vi "Live Capture Functional Stack.7.64bit.vi"() -> ()   [LabVIEW 2014]
uses:
  subvis/Stack Track.ctl
  subvis/Stack_State.ctl
  CameraControlTypeDef.ctl
  Desktop/camtiff/ctiff.llb/__CTIFFNewFileAndStyleUINT16.vi
  Desktop/camtiff/ctiff.llb/__CTIFFAddNewPageUINT16.vi
panel:
  in  "Capture Mode":bool
  out "Record Ready":bool
  in  "Stacks":dbl=1.0
  in  "Time Lapse":bool
  out "Stack Frames":i32=100
  in  "Stack Frames":i32=100
  in  "Temp":path=path "C:/temp.tmp"
  in  "Frames":i32=100
  in  "HardDisk Record":bool
  in  "Internal Line Interval":dbl
  in  "Slit Width / Lines":sgl=150.0
  in  "Camera Readout Mode":u16(ring)=12 items=["Full Frame"=1, "Slit Scanning"=12]
  in  "Readout Direction":sgl(ring)=1.0 items=["Forward"=1, "Backward"=2]
  in  "Trigger Mode":sgl(ring)=1.0 items=["Normal"=1, "Start "=6]
  in  "Trigger Source":sgl(ring)=2.0 items=["Internal"=1, "External"=2]
  out "State":T1=enum."Start Sequence"
  out "Image":u16[][](graph)
  out "Saving":bool
  in  "AutoIncrement":bool=TRUE
  in  "Path":path=path "C:/Users/spim/Desktop/Craig Cap/temp/a.tiff"
  in  "Frames":i32=100
  out "Frame Index":i32
  out "error out":errorcluster
  in  "stop":bool
  in  "Ram Record":bool
  out "Total Frames":i32
  out "Elapsed Time":u32
  out "Software FPS":dbl
  out "Camera FPS":dbl
  in  "H Offset":i32 min=0 max=0 step=4
  in  "H Width":i32 min=0 max=2048 step=4
  out "SMD":dbl
  out "SHO":i32
  in  "V Offset":i32 min=0 max=0 step=4
  in  "V Width":i32 min=0 max=2048 step=4
  in  "Binning":u16(ring) items=["1x1"=1, "2x2"=2, "4x4"=4]
  out "SHW":i32
  out "SVO":i32
  out "SVW":i32
  in  "Scan Mode":dbl min=0.0 max=2.0 step=1.0
  in  "Exposure":dbl min=0.0 max=10.000004210526315 step=1e-08
  out "EXP":dbl
  out "Camera Model":string
  out "Camera Version":string
  out "Camera Serial":string
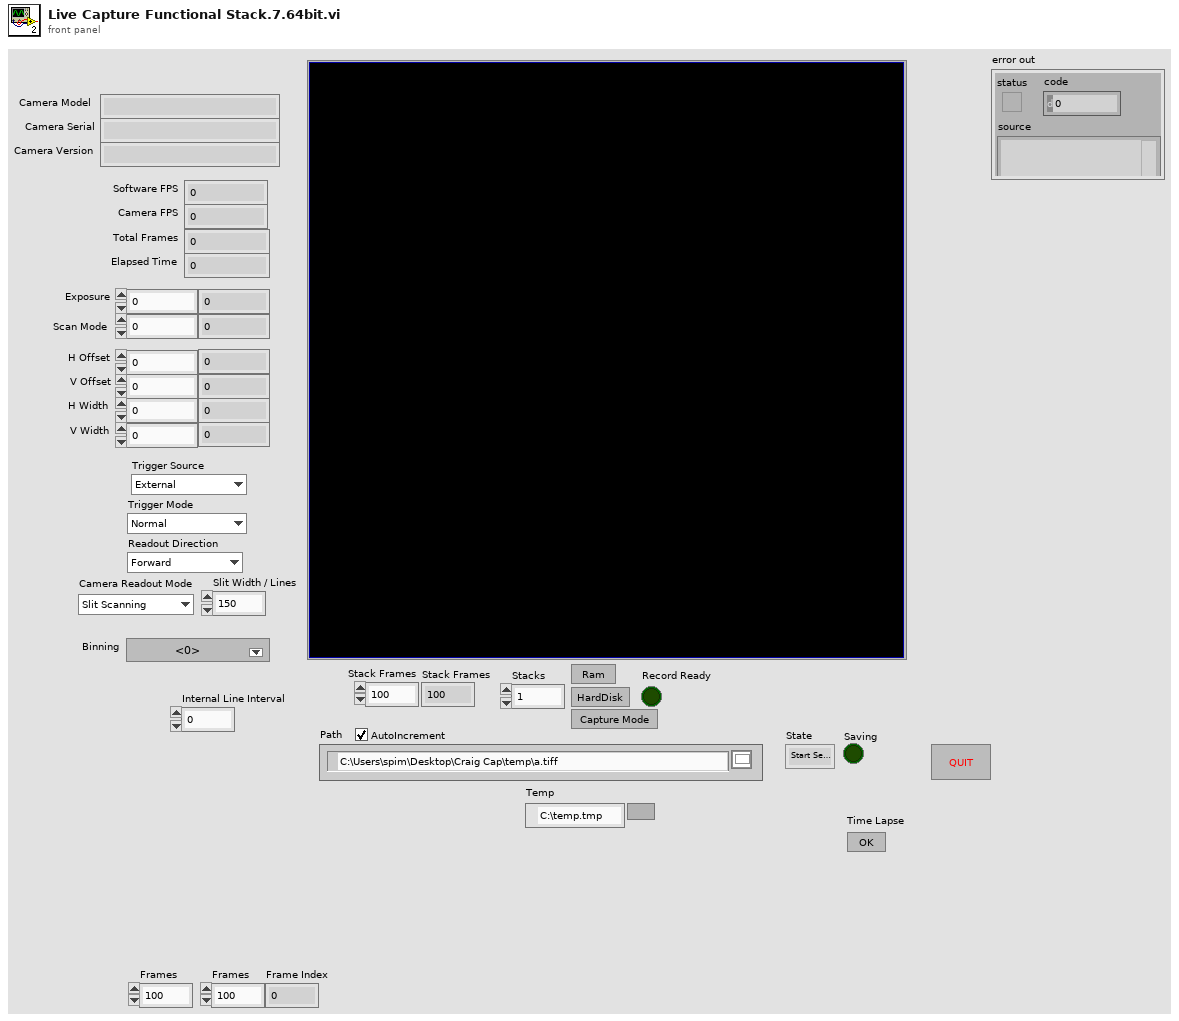
[diagram p1: front panel]
types:
  T1 = typedef "Stack Track.ctl" = enum16{"Idle", "Start Sequence", "Read Disk", "STOP", "Collecting", "End"}
  T2 = typedef "CameraControlTypeDef.ctl" = enum16{"IntervalLineInt", "Ram Record", "HardDisk Record", "Disengage Update", "Update", "Idle", "ROI", "Binning", "Scan Mode", "Trigger Mode", "Readout Mode", "Readout Direction", "Preview"}
  T3 = typedef "Stack_State.ctl" = cluster{"State":T1, "Stack Number":i32, "Image":u16[][], "Stacks":i32}
  T4 = enum8{"Enabled", "Disabled", "Disabled and Grayed Out"}
  T5 = cluster{"Model":string, "Camera ID":string, "Firmware":string}
  T6 = cluster{"Value":i32, "Minimum":i32, "Maximum":i32, "Increment":i32}
  T7 = cluster{"height":u32, "width":u32, "datatype":u32}
  T8 = cluster{"H Offset":i32, "V Offset":i32, "H Width":i32, "V Width":i32}
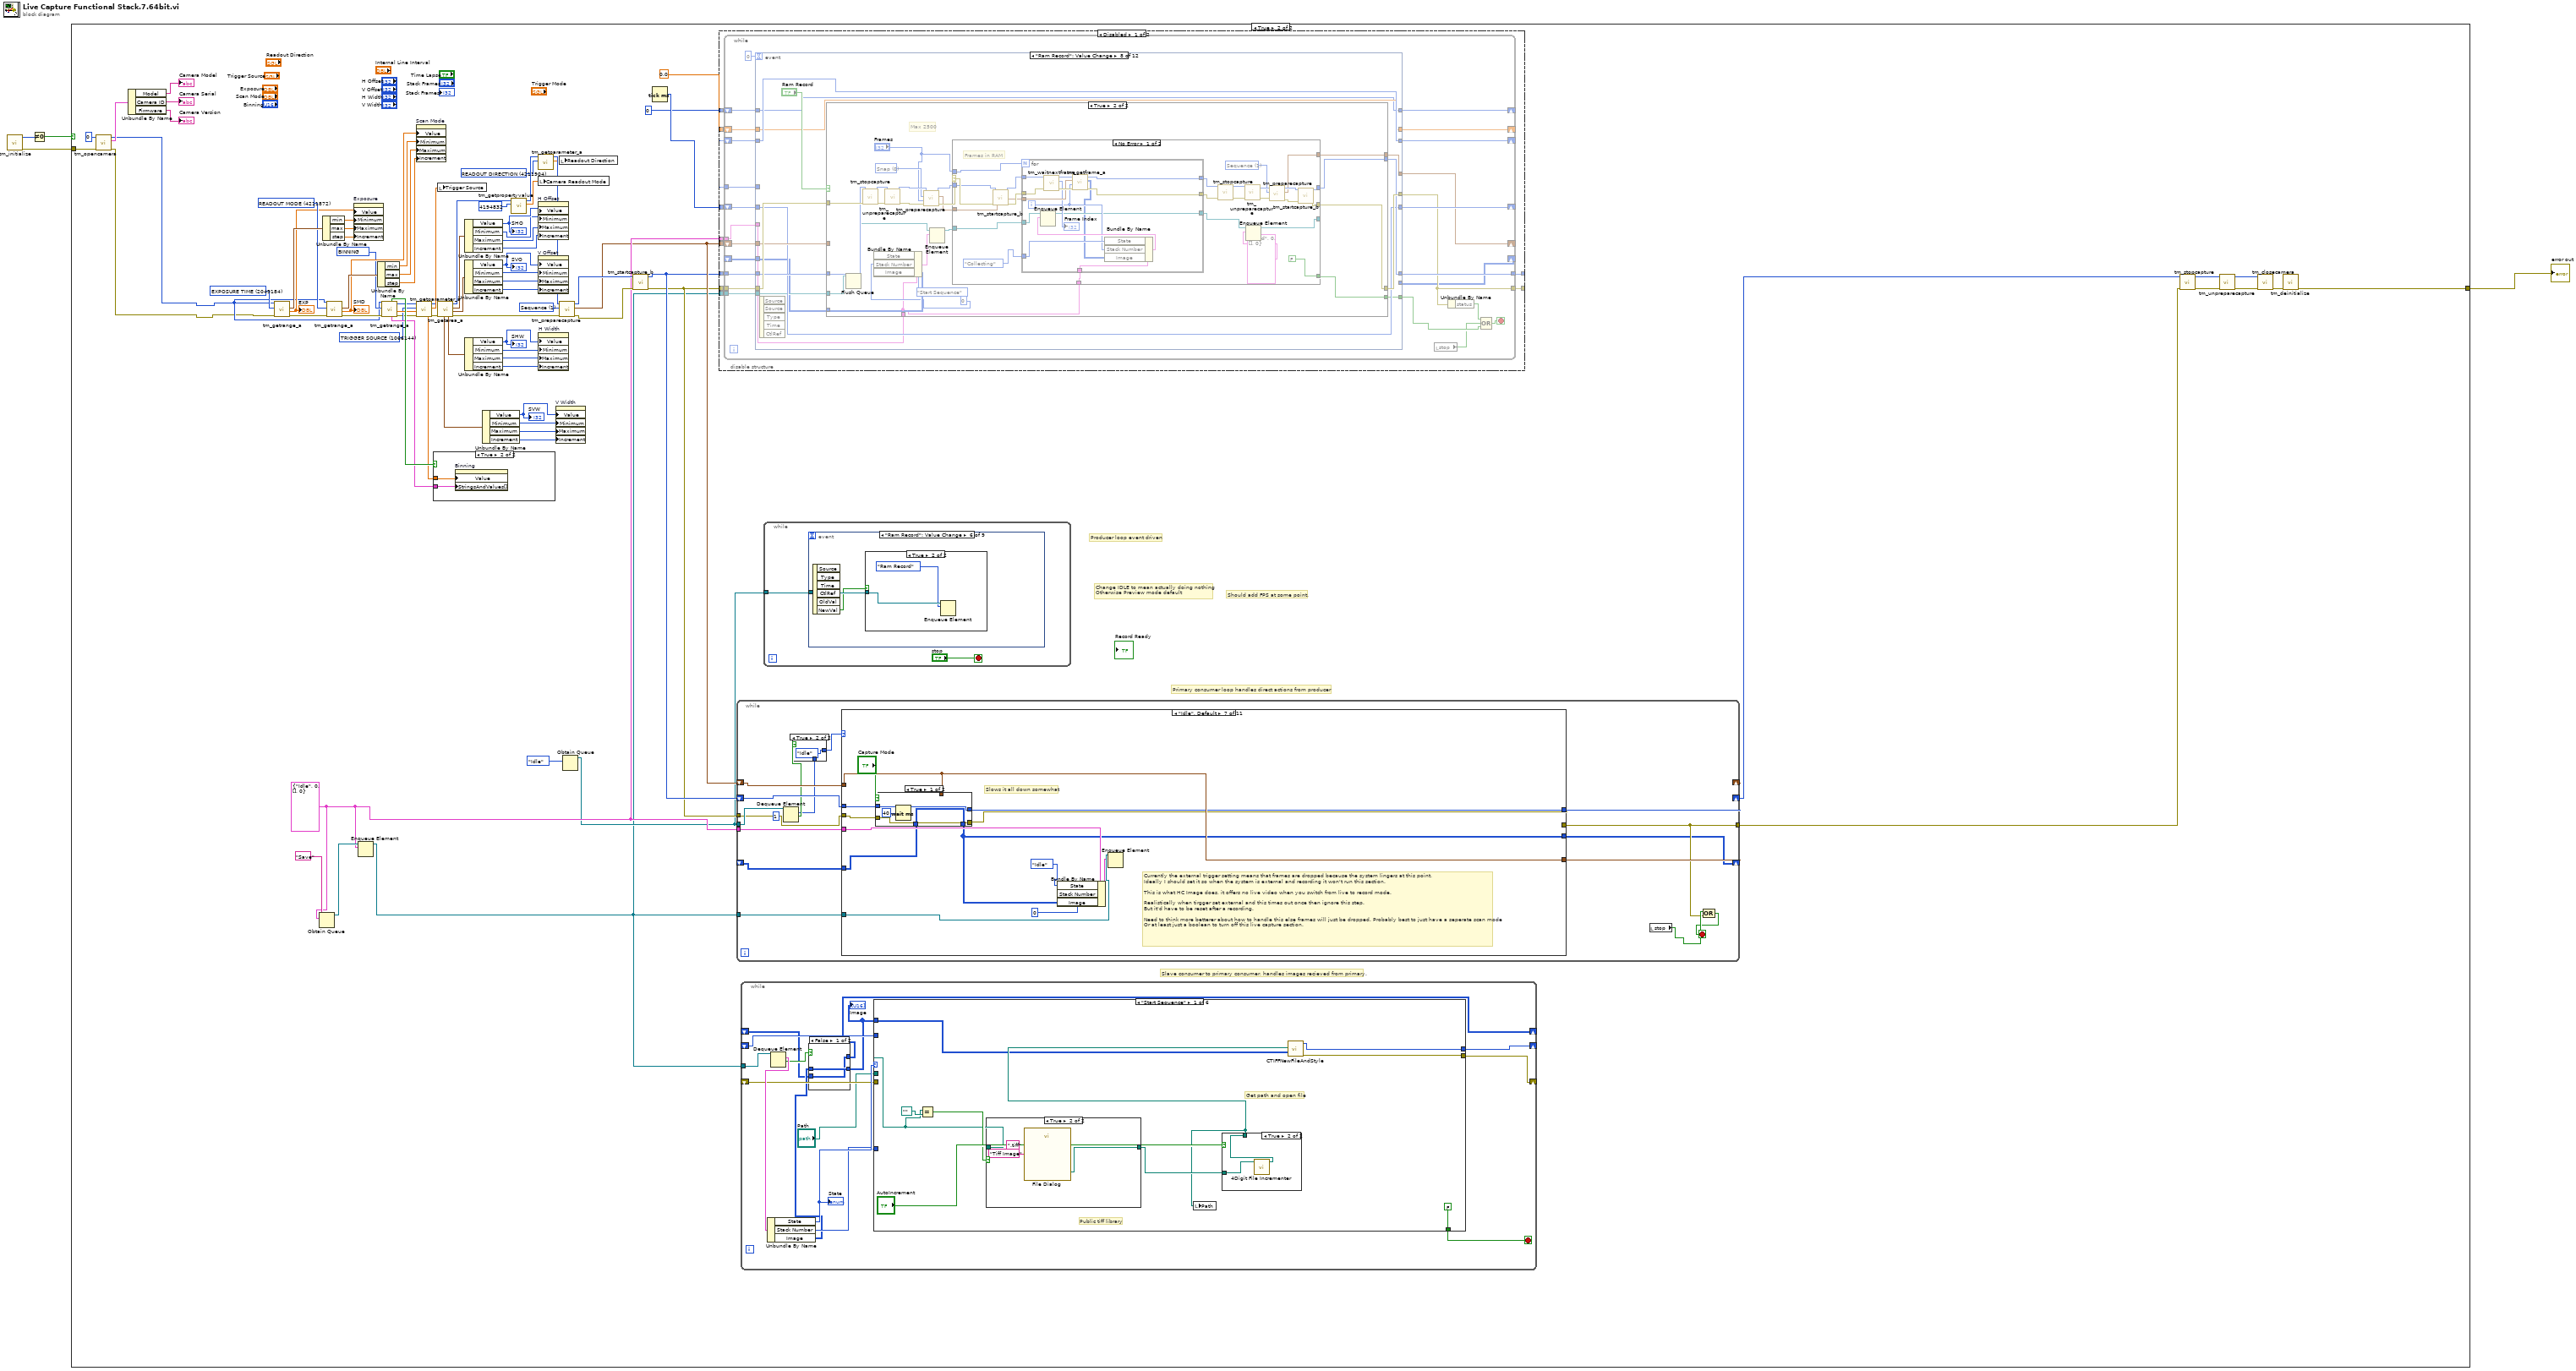
[diagram p0: block diagram]
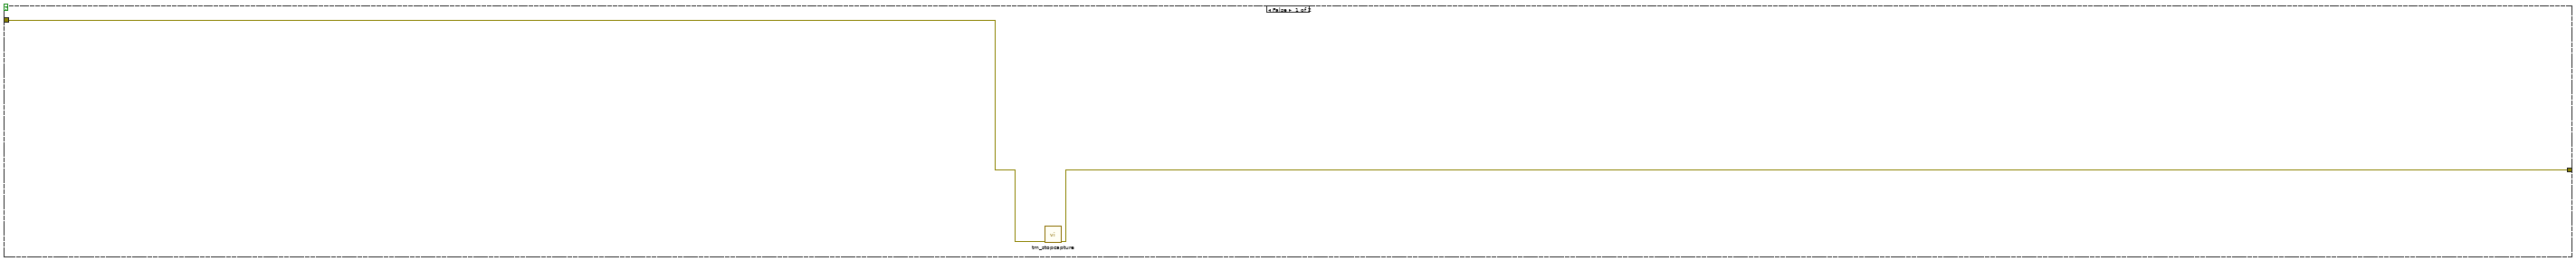
[diagram p2: hidden frame]
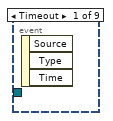
[diagram p3: hidden frame]
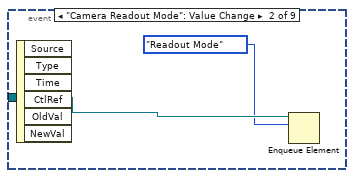
[diagram p4: hidden frame]
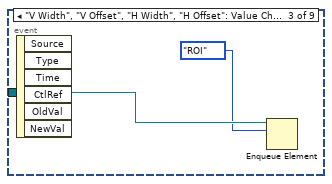
[diagram p5: hidden frame]
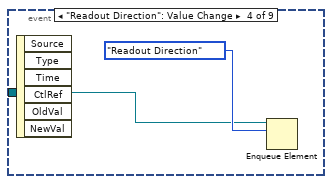
[diagram p6: hidden frame]
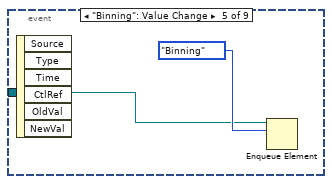
[diagram p7: hidden frame]
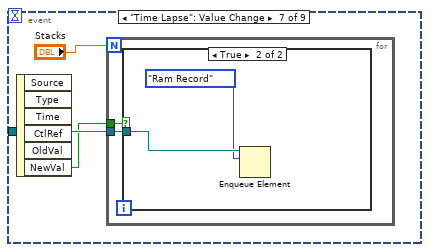
[diagram p9: hidden frame]
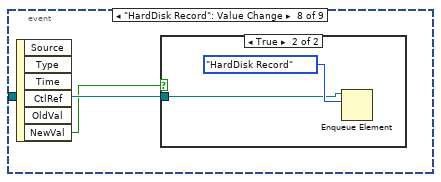
[diagram p11: hidden frame]
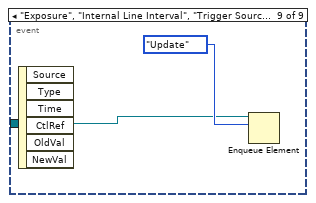
[diagram p13: hidden frame]
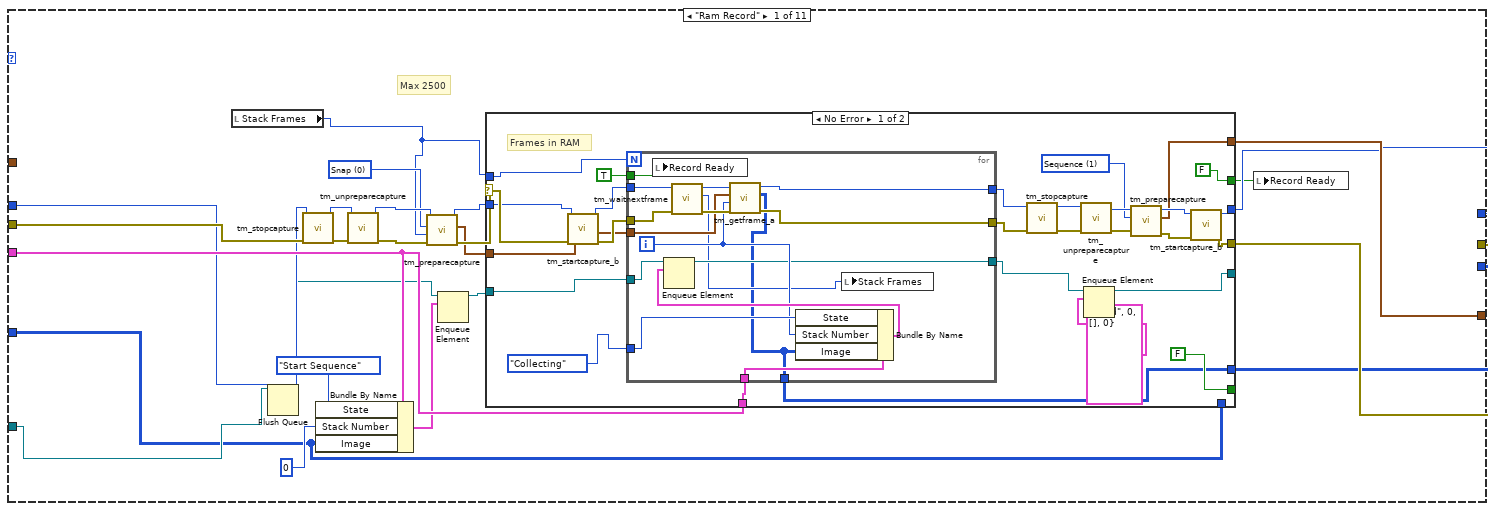
[diagram p15: hidden frame]
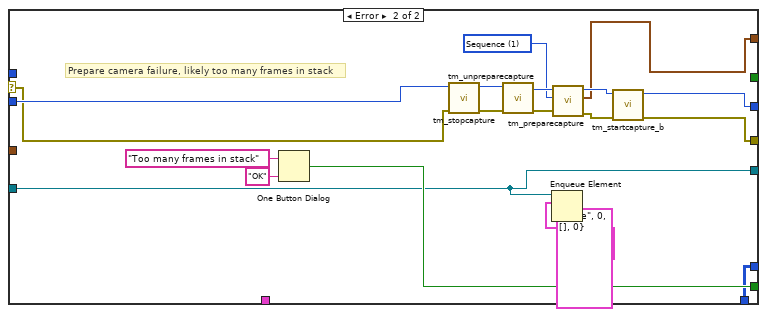
[diagram p16: hidden frame]
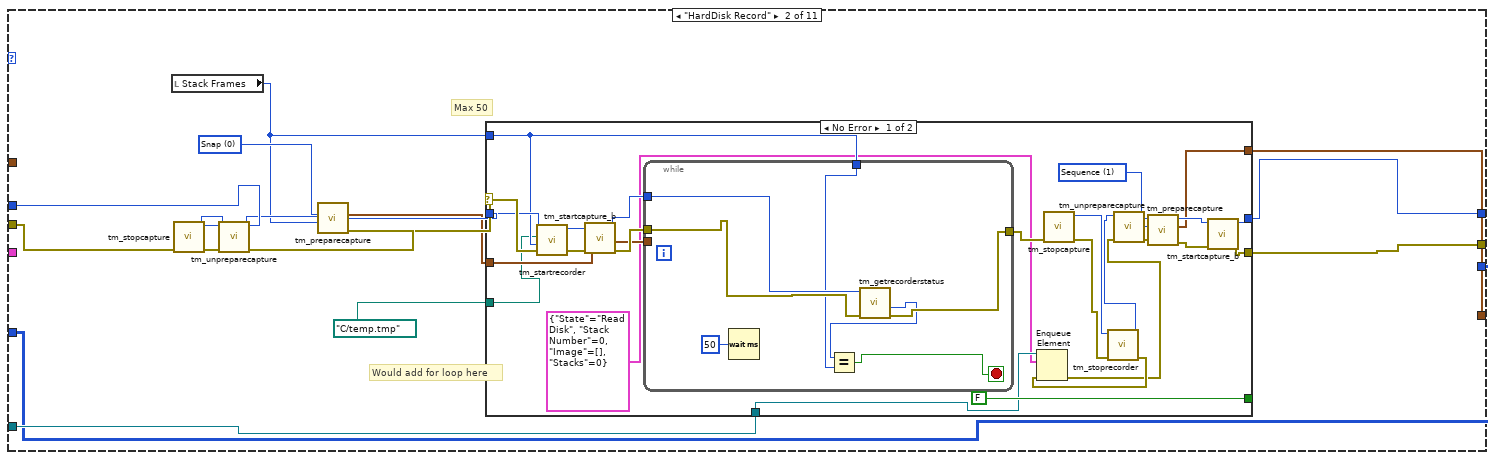
[diagram p17: hidden frame]
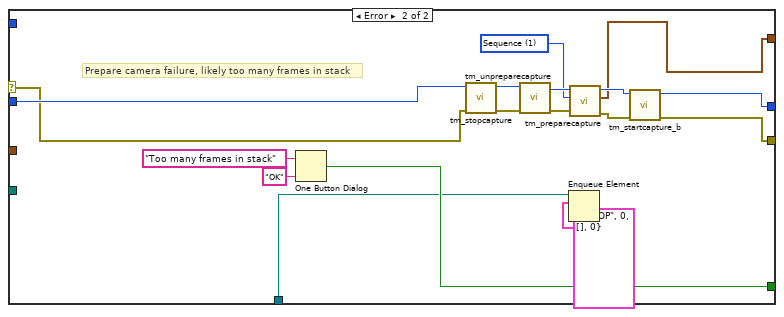
[diagram p18: hidden frame]
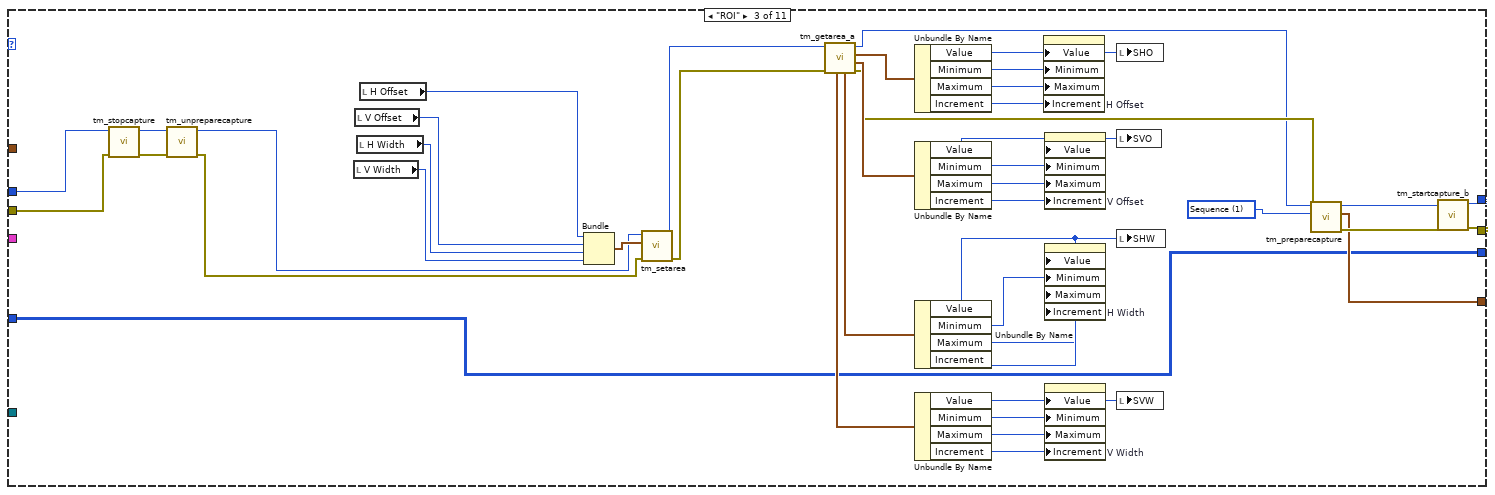
[diagram p19: hidden frame]
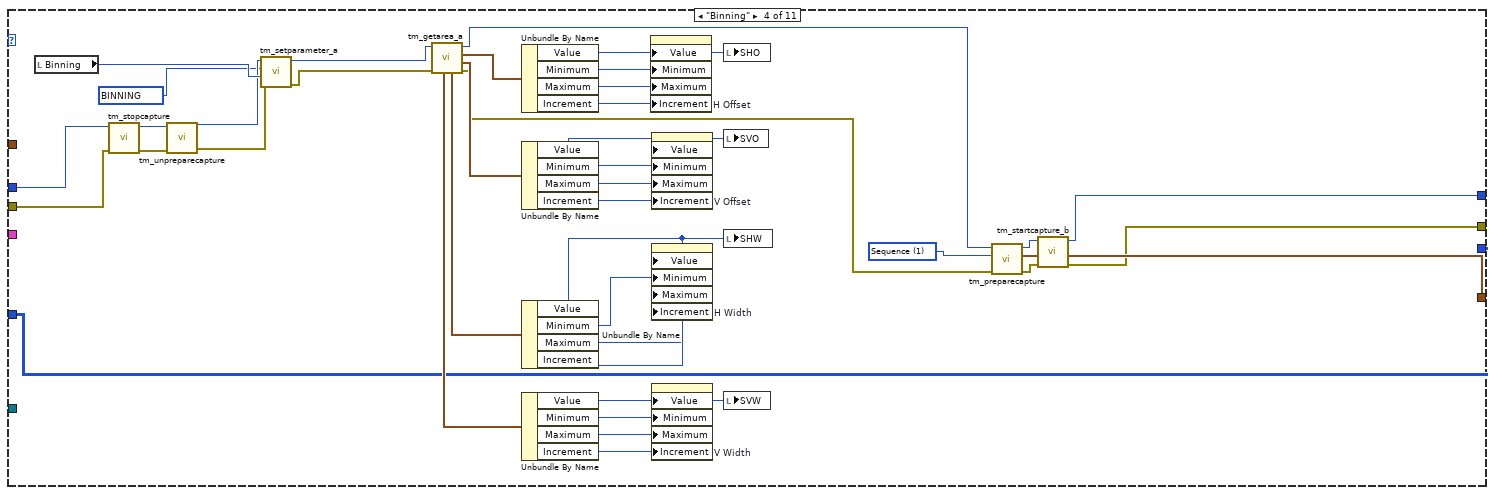
[diagram p20: hidden frame]
diagram:
  n1 = call <userlib>:"tm_initialize.vi"() -> ("error out"=w2:errorcluster, "Number Of Cameras"=w1:u32)  [unwired: 8 in, 2 out]
  n2 = Not Equal To 0?(x=w1) -> (x != 0?=w4:bool)
  n3 = case shown="True" w4 {
    tunnel: [w5 w86] -> w3
    tunnel: w2 -> [w6 w89]
    frame False {
      n4 = call <userlib>:"tm_stopcapture.vi"("error in (no error)"=w6) -> ("error out"=w5:errorcluster)  [unwired: 9 in, 1 out]
    }
    frame True {
      w22 = u32 4211904 items=["SENSOR MODE"=4212128, "CCD MODE"=4212384, "READOUT MODE"=4211872, "ACTIVE VIEW INDEX"=4343136, "BITS PER CHANNEL"=4342976, "IMAGE PIXEL TYPE"=4343296, "BINNING"=4215968, "EXPOSURE TIME"=2049184, "CONTRAST GAIN"=3163312, "CONTRAST OFFSET"=3163328, "LIGHT MODE"=2114720, "SENSITIVITY"=2114992, "PHOTON IMAGING MODE"=2115200, "HIGH DYNAMIC RANGE MODE"=3163360, "WHITE BALANCE"=3163568, "TEMPERATURE"=2115232, "TEMPERATURE TARGET"=2115264, "SENSOR COOLER FAN"=2115296, "LINEBUNDLE HEIGHT"=4212192, "MECHANICAL SHUTTER"=2115488, "BACK FOCUS POSITION"=8422304, "TRIGGER CONNECTOR"=1066432, "TRIGGER SOURCE"=1066144, "OUTPUT TRIGGER SOURCE"=1852576, "TRIGGER GLOBAL EXPOSURE"=2049680, "FIRST TRIGGER BEHAVIOR"=2049696, "CHANNEL SYNC"=1852352, "READOUT DIRECTION"=4211904, "PRE HSYNC COUNT"=1852704] ("Parameter")
      w32 = u32 1066144 items=["SENSOR MODE"=4212128, "CCD MODE"=4212384, "READOUT MODE"=4211872, "ACTIVE VIEW INDEX"=4343136, "BITS PER CHANNEL"=4342976, "IMAGE PIXEL TYPE"=4343296, "BINNING"=4215968, "EXPOSURE TIME"=2049184, "CONTRAST GAIN"=3163312, "CONTRAST OFFSET"=3163328, "LIGHT MODE"=2114720, "SENSITIVITY"=2114992, "PHOTON IMAGING MODE"=2115200, "HIGH DYNAMIC RANGE MODE"=3163360, "WHITE BALANCE"=3163568, "TEMPERATURE"=2115232, "TEMPERATURE TARGET"=2115264, "SENSOR COOLER FAN"=2115296, "LINEBUNDLE HEIGHT"=4212192, "MECHANICAL SHUTTER"=2115488, "BACK FOCUS POSITION"=8422304, "TRIGGER CONNECTOR"=1066432, "TRIGGER SOURCE"=1066144, "OUTPUT TRIGGER SOURCE"=1852576, "TRIGGER GLOBAL EXPOSURE"=2049680, "FIRST TRIGGER BEHAVIOR"=2049696, "CHANNEL SYNC"=1852352, "READOUT DIRECTION"=4211904, "PRE HSYNC COUNT"=1852704] ("Parameter")
      w15 = T3 {"State"=enum."Idle", "Stack Number"=0, "Image"=[], "Stacks"=0} ("input cluster")
      w37 = u32 2049184 items=["BINNING"=4215968, "BITS PER CHANNEL"=4342976, "ACTIVE VIEW INDEX"=4343136, "CCD MODE"=4212384, "SENSOR MODE"=4212128, "READOUT MODE"=4211872, "EXPOSURE TIME"=2049184, "CONTRAST GAIN"=3163312, "CONTRAST OFFSET"=3163328, "LIGHT MODE"=2114720, "SENSITIVITY"=2114992, "WHITE BALANCE"=3163568, "PHOTON IMAGING MODE"=2115200, "HIGH DYNAMIC RANGE MODE"=3163360, "TRIGGER SOURCE"=1066144, "TRIGGER ACTIVE"=1066160, "TRIGGER MODE"=1066400, "TRIGGER POLARITY"=1066416, "TRIGGER GLOBAL EXPOSURE"=2049680, "FIRST TRIGGER BEHAVIOR"=2049696, "TRIGGER TIMES"=1066448, "OUTPUT TRIGGER POLARITY"=1852592, "OUTPUT TRIGGER DELAY"=1852624, "OUTPUT TRIGGER PERIOD"=1852640, "TEMPERATURE"=2115232, "TEMPERATURE TARGET"=2115264, "SENSOR COOLER FAN"=2115296, "MECHANICAL SHUTTER"=2115488, "BACK FOCUS POSITION"=8422304, "FRAMEBUNDLE MODE"=4346784, "FRAMEBUNDLE NUMBER"=4346800, "LINEBUNDLE HEIGHT"=4212192, "TRIGGER CONNECTOR"=1066432, "IMAGE PIXEL TYPE"=4343296, "OUTPUT TRIGGER KIND"=1852656, "READOUT DIRECTION"=4211904, "CHANNEL SYNC"=1852352] ("Parameter")
      w38 = u32 4211872 items=["BINNING"=4215968, "BITS PER CHANNEL"=4342976, "ACTIVE VIEW INDEX"=4343136, "CCD MODE"=4212384, "SENSOR MODE"=4212128, "READOUT MODE"=4211872, "EXPOSURE TIME"=2049184, "CONTRAST GAIN"=3163312, "CONTRAST OFFSET"=3163328, "LIGHT MODE"=2114720, "SENSITIVITY"=2114992, "WHITE BALANCE"=3163568, "PHOTON IMAGING MODE"=2115200, "HIGH DYNAMIC RANGE MODE"=3163360, "TRIGGER SOURCE"=1066144, "TRIGGER ACTIVE"=1066160, "TRIGGER MODE"=1066400, "TRIGGER POLARITY"=1066416, "TRIGGER GLOBAL EXPOSURE"=2049680, "FIRST TRIGGER BEHAVIOR"=2049696, "TRIGGER TIMES"=1066448, "OUTPUT TRIGGER POLARITY"=1852592, "OUTPUT TRIGGER DELAY"=1852624, "OUTPUT TRIGGER PERIOD"=1852640, "TEMPERATURE"=2115232, "TEMPERATURE TARGET"=2115264, "SENSOR COOLER FAN"=2115296, "MECHANICAL SHUTTER"=2115488, "BACK FOCUS POSITION"=8422304, "FRAMEBUNDLE MODE"=4346784, "FRAMEBUNDLE NUMBER"=4346800, "LINEBUNDLE HEIGHT"=4212192, "TRIGGER CONNECTOR"=1066432, "IMAGE PIXEL TYPE"=4343296, "OUTPUT TRIGGER KIND"=1852656, "READOUT DIRECTION"=4211904, "CHANNEL SYNC"=1852352] ("Parameter")
      w39 = u32 4215968 items=["BINNING"=4215968, "BITS PER CHANNEL"=4342976, "ACTIVE VIEW INDEX"=4343136, "CCD MODE"=4212384, "SENSOR MODE"=4212128, "READOUT MODE"=4211872, "EXPOSURE TIME"=2049184, "CONTRAST GAIN"=3163312, "CONTRAST OFFSET"=3163328, "LIGHT MODE"=2114720, "SENSITIVITY"=2114992, "WHITE BALANCE"=3163568, "PHOTON IMAGING MODE"=2115200, "HIGH DYNAMIC RANGE MODE"=3163360, "TRIGGER SOURCE"=1066144, "TRIGGER ACTIVE"=1066160, "TRIGGER MODE"=1066400, "TRIGGER POLARITY"=1066416, "TRIGGER GLOBAL EXPOSURE"=2049680, "FIRST TRIGGER BEHAVIOR"=2049696, "TRIGGER TIMES"=1066448, "OUTPUT TRIGGER POLARITY"=1852592, "OUTPUT TRIGGER DELAY"=1852624, "OUTPUT TRIGGER PERIOD"=1852640, "TEMPERATURE"=2115232, "TEMPERATURE TARGET"=2115264, "SENSOR COOLER FAN"=2115296, "MECHANICAL SHUTTER"=2115488, "BACK FOCUS POSITION"=8422304, "FRAMEBUNDLE MODE"=4346784, "FRAMEBUNDLE NUMBER"=4346800, "LINEBUNDLE HEIGHT"=4212192, "TRIGGER CONNECTOR"=1066432, "IMAGE PIXEL TYPE"=4343296, "OUTPUT TRIGGER KIND"=1852656, "READOUT DIRECTION"=4211904, "CHANNEL SYNC"=1852352] ("Parameter")
      w84 = 1 items=["Snap", "Sequence"] ("Capture mode")
      # "Change IDLE to mean actually doing nothing\nOtherwise Preview mode default"
      # "Slave consumer to primary consumer, handles images recieved from primary."
      # "Primary consumer loop handles direct actions from producer"
      # "Producer loop event driven"
      # "Should add FPS at some point."
      n5 = call <userlib>:"tm_opencamera.vi"("error in (no error)"=w89, "Camera Index"=u32 0) -> ("error out"=w16:errorcluster, "Camera Details"=w51:T5, "Handle out"=w17:u32)  [unwired: 7 in]
      n6 = Unbundle By Name(w51) -> ("Model"=→"Camera Model":string, "Camera ID"=→"Camera Serial":string, "Firmware"=→"Camera Version":string)
      n7 = call <userlib>:"tm_getrange_a.vi"("error in (no error)"=w16, "Parameter"=w37, "Handle in"=w17) -> ("error out"=w46:errorcluster, "default"=w35:dbl, "Range"=w47:cluster{"min":dbl, "max":dbl, "step":dbl})  [unwired: 2 in, 4 out]
      "EXP" <- w35
      n8 = Obtain Queue(name (unnamed)="Save", element data type=w15) -> (queue out=w19:refnum<queue>)  [unwired: 3 in, 2 out]
      n9 = Unbundle By Name(w47) -> ("min"=w82:dbl, "max"=w81:dbl, "step"=w80:dbl)
      n10 = call <userlib>:"tm_getrange_a.vi"("error in (no error)"=w46, "Parameter"=w38, "Handle in"=w17) -> ("error out"=w43:errorcluster, "default"=w44:dbl, "Range"=w45:cluster{"min":dbl, "max":dbl, "step":dbl})  [unwired: 2 in, 4 out]
      "SMD" <- w44
      n11 = property on="Exposure" class="DigNum (strict)"("Value"=w35, "Minimum"=w82, "Maximum"=w81, "Increment"=w80) -> ()  [unwired: 2 in, 2 out]
      n12 = Enqueue Element(queue=w19, element=w15) -> (queue out=w9:refnum<queue>)  [unwired: 2 in, 2 out]
      n13 = Unbundle By Name(w45) -> ("min"=w79:dbl, "max"=w78:dbl, "step"=w77:dbl)
      n14 = call <userlib>:"tm_getrange_a.vi"("error in (no error)"=w43, "Parameter"=w39, "Handle in"=w17) -> ("error out"=w29:errorcluster, "default"=w41:dbl, "Handle out"=w31:u32, "Value Names"=w40:cluster{"Name":string, "Value":dbl}[], "Writable"=w42:bool)  [unwired: 2 in, 2 out]
      n15 = property on="Scan Mode" class="DigNum (strict)"("Value"=w44, "Minimum"=w79, "Maximum"=w78, "Increment"=w77) -> ()  [unwired: 2 in, 2 out]
      n16 = call <userlib>:"tm_getparameter_a.vi"("error in (no error)"=w29, "Parameter"=w32, "Handle in"=w31) -> ("error out"=w28:errorcluster, "Value out"=w33:dbl, "Handle out"=w30:u32)  [unwired: 6 in]
      n17 = case shown="True" w42 {
        tunnel: w40 -> [_ w1109]
        tunnel: w41 -> [_ w1108]
        frame False {
        }
        frame True {
          n18 = property on="Binning" class="Ring (strict)"("Value"=w1108, "StringsAndValues[]"=w1109) -> ()  [unwired: 2 in, 2 out]
        }
      }
      n19 = local write "Trigger Source"(w33) -> ()
      n20 = call <userlib>:"tm_getarea_a.vi"("error in (no error)"=w28, "Handle in"=w30) -> ("error out"=w34:errorcluster, "V Offset"=w76:T6, "H Offset"=w57:T6, "Handle out"=w25:u32, "H Width"=w75:T6, "V Width"=w74:T6)  [unwired: 4 in]
      n21 = Unbundle By Name(w57) -> ("Value"=w56:i32, "Minimum"=w55:i32, "Maximum"=w54:i32, "Increment"=w53:i32)
      "SHO" <- w56
      n22 = Unbundle By Name(w76) -> ("Value"=w64:i32, "Minimum"=w73:i32, "Maximum"=w72:i32, "Increment"=w71:i32)
      "SVO" <- w64
      n23 = Unbundle By Name(w75) -> ("Value"=w63:i32, "Minimum"=w70:i32, "Maximum"=w69:i32, "Increment"=w68:i32)
      "SHW" <- w63
      n24 = Unbundle By Name(w74) -> ("Value"=w62:i32, "Minimum"=w67:i32, "Maximum"=w66:i32, "Increment"=w65:i32)
      "SVW" <- w62
      n25 = call <userlib>:"tm_getpropertyvalue.vi"("Property ID"=u32 4194832, "Handle in"=w25) -> ("Value in"=w26:sgl, "Handle out"=w24:u32)  [unwired: 7 in, 1 out]
      n26 = call <userlib>:"tm_getparameter_a.vi"("Parameter"=w22, "Handle in"=w24) -> ("Value out"=w21:dbl, "Handle out"=w23:u32)  [unwired: 7 in, 1 out]
      n27 = local write "Camera Readout Mode"(w26) -> ()
      n28 = property on="H Offset" class="DigNum (strict)"("Value"=w56, "Minimum"=w55, "Maximum"=w54, "Increment"=w53) -> ()  [unwired: 2 in, 2 out]
      n29 = property on="V Offset" class="DigNum (strict)"("Value"=w64, "Minimum"=w73, "Maximum"=w72, "Increment"=w71) -> ()  [unwired: 2 in, 2 out]
      n30 = property on="H Width" class="DigNum (strict)"("Value"=w63, "Minimum"=w70, "Maximum"=w69, "Increment"=w68) -> ()  [unwired: 2 in, 2 out]
      n31 = property on="V Width" class="DigNum (strict)"("Value"=w62, "Minimum"=w67, "Maximum"=w66, "Increment"=w65) -> ()  [unwired: 2 in, 2 out]
      n32 = local write "Readout Direction"(w21) -> ()
      n33 = call <userlib>:"tm_preparecapture.vi"("error in (no error)"=w34, "Capture mode"=w84, "Handle in"=w23) -> ("error out"=w18:errorcluster, "Buffer Info"=w14:T7, "Handle out"=w20:u32)  [unwired: 5 in, 1 out]
      n34 = Obtain Queue(element data type=CameraControlTypeDef."Idle" ("Enum")) -> (queue out=w10:refnum<queue>)  [unwired: 4 in, 2 out]
      n35 = call <userlib>:"tm_startcapture_b.vi"("error in (no error)"=w18, "Handle in"=w20) -> ("error out"=w12:errorcluster, "Handle out"=w13:u32)  [unwired: 8 in]
      n36 = Tick Count (ms)() -> (millisecond timer value=w83:u32)
      n37 = disable-structure shown="Disabled" {
        disable-tunnel: 0.0 -> [w525 _]
        disable-tunnel: w83 -> [w524 _]
        disable-tunnel: 0 -> [w523 _]
        disable-tunnel: [w522 _] -> _
        disable-tunnel: [w521 _] -> _
        disable-tunnel: w15 -> [w520 _]
        disable-tunnel: w14 -> [w519 _]
        disable-tunnel: w13 -> [w518 _]
        disable-tunnel: w12 -> [w517 _]
        disable-tunnel: w9 -> [w516 _]
        frame Disabled {
          n38 = while {
            tunnel: w517 -> [w539]
            tunnel: [w537] -> w521
            tunnel: [w536] -> w522
            shift-right: [w546] -> _
            shift-left: w524 -> [w544]
            shift-right: [w547] -> _
            shift-left: w525 -> [w545]
            shift-right: [w538] -> _
            shift-left: w524 -> [w542]
            tunnel: w518 -> [w540]
            tunnel: w524 -> [w543]
            shift-right: [w535] -> _
            shift-left: w519 -> [w541]
            shift-right: [w533] -> _
            shift-left: w523 -> [w534]
            tunnel: w516 -> [w532]
            shift-right: [w530] -> _
            shift-left: _ -> [w529]
            tunnel: w520 -> [w528]
            stop <- w548 stop-if-true
            n39 = event shown="[7] \"Ram Record\": Value Change" {
              selector: _ -> [_ _ _ _ _ _ _ _ _ _ _ _]
              dyn-events: _ -> [_ _ _ _ _ _ _ _ _ _ _ _]
              timeout: 0 -> [_ _ _ _ _ _ _ _ _ _ _ _]
              tunnel: [w559 w628 w642 w655 w674 w694 w716 w744 w841 w935 w971 w1016] -> w547
              tunnel: [w558 w629 w643 w656 w675 w695 w717 w745 w842 w936 w972 w1017] -> w546
              tunnel: w545 -> [w570 w628 w642 w655 w674 w694 w716 w744 w841 w935 w971 w1016]
              tunnel: w544 -> [w561 w629 w643 w656 w675 w695 w717 w745 w842 w936 w972 w1017]
              tunnel: w543 -> [w566 _ _ _ _ _ _ _ _ _ _ _]
              tunnel: w542 -> [w571 w630 w644 w657 w676 w696 w718 w740 w837 w937 w979 w1024]
              tunnel: w541 -> [w565 w627 w641 w654 _ w693 _ w741 w838 _ _ _]
              tunnel: w540 -> [w573 w623 w636 w650 w669 w687 w709 w748 w845 w932 w948 w986]
              tunnel: w539 -> [w572 w625 w632 w651 w668 w690 w708 w749 w846 w931 w947 w985]
              tunnel: [w569 w630 w644 w657 w676 w696 w718 w740 w837 w937 w979 w1024] -> w538
              tunnel: [w568 w620 w639 w647 w660 w680 w699 w746 w843 w926 w974 w1019] -> w537
              tunnel: [w567 w619 w638 w646 w659 w679 w697 w747 w844 w927 w975 w1020] -> w536
              tunnel: [w564 w627 w641 w654 w663 w693 w704 w742 w839 w925 w973 w1018] -> w535
              tunnel: w534 -> [w556 w626 w640 w653 w673 w692 w715 w743 w840 w924 w944 w980]
              tunnel: [w555 w626 w640 w653 w673 w692 w715 w743 w840 w924 w944 w980] -> w533
              tunnel: w532 -> [w550 _ _ _ _ _ _ w739 w836 _ _ _]
              tunnel: [_ _ _ _ _ _ _ w738 w835 _ _ _] -> w531
              tunnel: w528 -> [w553 _ _ _ _ _ _ w736 _ _ _ _]
              tunnel: [w552 _ _ _ _ _ _ _ _ _ _ _] -> w530
              tunnel: w529 -> [w551 _ _ _ _ _ _ w737 _ _ _ _]
              event Timeout {
                n40 = event-data() -> ()  [unwired: 1 in, 2 out]
                n41 = call <userlib>:"tm_waitnextframe.vi"("error in (no error)"=w572, "Handle in"=w573) -> ("error out"=w576:errorcluster, "Frame Count"=w557:i32, "Frame Index"=w575:i32, "Handle out"=w577:u32)  [unwired: 6 in]
                "Total Frames" <- w557
                n42 = Tick Count (ms)() -> (millisecond timer value=w563:u32)
                n43 = Increment(x=w570) -> (x+1=w560:dbl)
                n44 = Subtract(x=w563, y=w566) -> (x-y=→"Elapsed Time":u32)
                n45 = Add(x=w561, y=u32 1000) -> (x+y=w581:u32)
                n46 = Less Or Equal?(x=w581, y=w563) -> (x <= y?=w562:bool)
                n47 = Add(x=w571, y=u32 50) -> (x+y=w579:u32)
                n48 = Less Or Equal?(x=w579, y=w563) -> (x <= y?=w554:bool)
                n49 = case shown="True" w562 {
                  tunnel: w561 -> [w584 w593]
                  tunnel: [w584 w590] -> w558
                  tunnel: w560 -> [w583 w596]
                  tunnel: w563 -> [_ w590]
                  tunnel: [w583 0.0] -> w559
                  tunnel: w557 -> [_ w585]
                  tunnel: w556 -> [w582 w588]
                  tunnel: [w582 w585] -> w555
                  frame False {
                  }
                  frame True {
                    n50 = Subtract(x=w590, y=w593) -> (x-y=w592:u32)
                    n51 = Subtract(x=w585, y=w588) -> (x-y=w586:i32)
                    n52 = To Double Precision Float(number=w592) -> (double precision float=w598:dbl)
                    n53 = Divide(x=w598, y=1000.0) -> (x/y=w589:dbl)
                    n54 = To Double Precision Float(number=w586) -> (double precision float=w587:dbl)
                    n55 = Divide(x=w587, y=w589) -> (x/y=→"Camera FPS":dbl)
                    n56 = Divide(x=w596, y=w589) -> (x/y=→"Software FPS":dbl)
                  }
                }
                n57 = case shown="True" w554 {
                  tunnel: w571 -> [w603 _]
                  tunnel: w563 -> [_ w616]
                  tunnel: [w603 w616] -> w569
                  tunnel: w577 -> [w602 w615]
                  tunnel: w565 -> [w600 w610]
                  tunnel: w576 -> [w601 w614]
                  tunnel: [w602 w613] -> w568
                  tunnel: [w601 w612] -> w567
                  tunnel: w575 -> [_ w611]
                  tunnel: [w600 w610] -> w564
                  tunnel: w550 -> [_ w609]
                  tunnel: w553 -> [_ w605]
                  tunnel: [w599 w604] -> w552
                  tunnel: w551 -> [w599 _]
                  frame False {
                  }
                  frame True {
                    n58 = call <userlib>:"tm_getframe_a.vi"("error in (no error)"=w614, "Frame Index"=w611, "Buffer Info"=w610, "Handle in"=w615) -> ("error out"=w612:errorcluster, "Data 16"=w604:u16[][], "Handle out"=w613:u32)  [unwired: 3 in, 2 out]
                    n59 = Bundle By Name(cluster=w605, "State"=Stack_Track."Idle", "Stack Number"=0, "Image"=w604) -> (w606:T3)
                    n60 = Enqueue Element(queue=w609, element=w606) -> ()  [unwired: 2 in, 3 out]
                  }
                }
              }
              event "Exposure": Value Change {
                w618 = u32 2049184 items=["SENSOR MODE"=4212128, "CCD MODE"=4212384, "READOUT MODE"=4211872, "ACTIVE VIEW INDEX"=4343136, "BITS PER CHANNEL"=4342976, "IMAGE PIXEL TYPE"=4343296, "BINNING"=4215968, "EXPOSURE TIME"=2049184, "CONTRAST GAIN"=3163312, "CONTRAST OFFSET"=3163328, "LIGHT MODE"=2114720, "SENSITIVITY"=2114992, "PHOTON IMAGING MODE"=2115200, "HIGH DYNAMIC RANGE MODE"=3163360, "WHITE BALANCE"=3163568, "TEMPERATURE"=2115232, "TEMPERATURE TARGET"=2115264, "SENSOR COOLER FAN"=2115296, "LINEBUNDLE HEIGHT"=4212192, "MECHANICAL SHUTTER"=2115488, "BACK FOCUS POSITION"=8422304, "TRIGGER CONNECTOR"=1066432, "TRIGGER SOURCE"=1066144, "OUTPUT TRIGGER SOURCE"=1852576, "TRIGGER GLOBAL EXPOSURE"=2049680, "FIRST TRIGGER BEHAVIOR"=2049696, "CHANNEL SYNC"=1852352, "READOUT DIRECTION"=4211904, "PRE HSYNC COUNT"=1852704] ("Parameter")
                n61 = event-data() -> ("NewVal"=w624:dbl)  [unwired: 1 in, 2 out]
                n62 = call <userlib>:"tm_setparameter_a.vi"("error in (no error)"=w625, "Value in"=w624, "Parameter"=w618, "Handle in"=w623) -> ("error out"=w622:errorcluster, "Handle out"=w621:u32)  [unwired: 6 in]
                n63 = call <userlib>:"tm_getparameter_a.vi"("error in (no error)"=w622, "Parameter"=w618, "Handle in"=w621) -> ("error out"=w619:errorcluster, "Value out"=w617:dbl, "Handle out"=w620:u32)  [unwired: 6 in]
                n64 = local write "EXP"(w617) -> ()
              }
              event "Internal Line Interval": Value Change {
                w631 = u32 4191424 items=["SENSOR MODE"=4212128, "CCD MODE"=4212384, "READOUT MODE"=4211872, "ACTIVE VIEW INDEX"=4343136, "BITS PER CHANNEL"=4342976, "IMAGE PIXEL TYPE"=4343296, "BINNING"=4215968, "EXPOSURE TIME"=2049184, "CONTRAST GAIN"=3163312, "CONTRAST OFFSET"=3163328, "LIGHT MODE"=2114720, "SENSITIVITY"=2114992, "PHOTON IMAGING MODE"=2115200, "HIGH DYNAMIC RANGE MODE"=3163360, "WHITE BALANCE"=3163568, "TEMPERATURE"=2115232, "TEMPERATURE TARGET"=2115264, "SENSOR COOLER FAN"=2115296, "LINEBUNDLE HEIGHT"=4212192, "MECHANICAL SHUTTER"=2115488, "BACK FOCUS POSITION"=8422304, "TRIGGER CONNECTOR"=1066432, "TRIGGER SOURCE"=1066144, "OUTPUT TRIGGER SOURCE"=1852576, "TRIGGER GLOBAL EXPOSURE"=2049680, "FIRST TRIGGER BEHAVIOR"=2049696, "CHANNEL SYNC"=1852352, "READOUT DIRECTION"=4211904, "PRE HSYNC COUNT"=1852704, "INTERNAL LINE SPEED"=4191408, "INTERNAL LINE INVERVAL"=4191424] ("Parameter")
                n65 = event-data() -> ("NewVal"=w635:dbl)  [unwired: 1 in, 2 out]
                n66 = call <userlib>:"tm_setparameter_a.vi"("error in (no error)"=w632, "Value in"=w635, "Parameter"=w631, "Handle in"=w636) -> ("error out"=w633:errorcluster, "Handle out"=w634:u32)  [unwired: 6 in]
                n67 = call <userlib>:"tm_getparameter_a.vi"("error in (no error)"=w633, "Parameter"=w631, "Handle in"=w634) -> ("error out"=w638:errorcluster, "Value out"=w637:dbl, "Handle out"=w639:u32)  [unwired: 6 in]
                n68 = local write "Internal Line Interval"(w637) -> ()
              }
              event "Trigger Source": Value Change {
                w652 = u32 1066144 items=["SENSOR MODE"=4212128, "CCD MODE"=4212384, "READOUT MODE"=4211872, "ACTIVE VIEW INDEX"=4343136, "BITS PER CHANNEL"=4342976, "IMAGE PIXEL TYPE"=4343296, "BINNING"=4215968, "EXPOSURE TIME"=2049184, "CONTRAST GAIN"=3163312, "CONTRAST OFFSET"=3163328, "LIGHT MODE"=2114720, "SENSITIVITY"=2114992, "PHOTON IMAGING MODE"=2115200, "HIGH DYNAMIC RANGE MODE"=3163360, "WHITE BALANCE"=3163568, "TEMPERATURE"=2115232, "TEMPERATURE TARGET"=2115264, "SENSOR COOLER FAN"=2115296, "LINEBUNDLE HEIGHT"=4212192, "MECHANICAL SHUTTER"=2115488, "BACK FOCUS POSITION"=8422304, "TRIGGER CONNECTOR"=1066432, "TRIGGER SOURCE"=1066144, "OUTPUT TRIGGER SOURCE"=1852576, "TRIGGER GLOBAL EXPOSURE"=2049680, "FIRST TRIGGER BEHAVIOR"=2049696, "CHANNEL SYNC"=1852352, "READOUT DIRECTION"=4211904, "PRE HSYNC COUNT"=1852704] ("Parameter")
                n69 = event-data() -> ("NewVal"=w645:sgl)  [unwired: 1 in, 3 out]
                n70 = call <userlib>:"tm_setparameter_a.vi"("error in (no error)"=w651, "Value in"=w645, "Parameter"=w652, "Handle in"=w650) -> ("error out"=w649:errorcluster, "Handle out"=w648:u32)  [unwired: 6 in]
                n71 = call <userlib>:"tm_getparameter_a.vi"("error in (no error)"=w649, "Parameter"=w652, "Handle in"=w648) -> ("error out"=w646:errorcluster, "Handle out"=w647:u32)  [unwired: 6 in, 1 out]
              }
              event "Trigger Mode": Value Change {
                w664 = 1 items=["Snap", "Sequence"] ("Capture mode")
                n72 = event-data() -> ("NewVal"=w658:sgl)  [unwired: 1 in, 4 out]
                n73 = call <userlib>:"tm_stopcapture.vi"("error in (no error)"=w668, "Handle in"=w669) -> ("error out"=w671:errorcluster, "Handle out"=w670:u32)  [unwired: 8 in]
                n74 = call <userlib>:"tm_unpreparecapture.vi"("error in (no error)"=w671, "Handle in"=w670) -> ("error out"=w667:errorcluster, "Handle out"=w666:u32)  [unwired: 8 in]
                n75 = call <userlib>:"tm_setpropertyvalue.vi"("error in (no error)"=w667, "Value in"=w658, "Property ID"=u32 1049104, "Handle in"=w666) -> ("error out"=w662:errorcluster, "Handle out"=w665:u32)  [unwired: 6 in]
                n76 = call <userlib>:"tm_preparecapture.vi"("Capture mode"=w664, "Handle in"=w665) -> ("Buffer Info"=w663:T7, "Handle out"=w661:u32)  [unwired: 6 in, 2 out]
                n77 = call <userlib>:"tm_startcapture_b.vi"("error in (no error)"=w662, "Handle in"=w661) -> ("error out"=w659:errorcluster, "Handle out"=w660:u32)  [unwired: 8 in]
              }
              event "Readout Direction": Value Change {
                w685 = 1 items=["Snap", "Sequence"] ("Capture mode")
                w678 = u32 4211904 items=["SENSOR MODE"=4212128, "CCD MODE"=4212384, "READOUT MODE"=4211872, "ACTIVE VIEW INDEX"=4343136, "BITS PER CHANNEL"=4342976, "IMAGE PIXEL TYPE"=4343296, "BINNING"=4215968, "EXPOSURE TIME"=2049184, "CONTRAST GAIN"=3163312, "CONTRAST OFFSET"=3163328, "LIGHT MODE"=2114720, "SENSITIVITY"=2114992, "PHOTON IMAGING MODE"=2115200, "HIGH DYNAMIC RANGE MODE"=3163360, "WHITE BALANCE"=3163568, "TEMPERATURE"=2115232, "TEMPERATURE TARGET"=2115264, "SENSOR COOLER FAN"=2115296, "LINEBUNDLE HEIGHT"=4212192, "MECHANICAL SHUTTER"=2115488, "BACK FOCUS POSITION"=8422304, "TRIGGER CONNECTOR"=1066432, "TRIGGER SOURCE"=1066144, "OUTPUT TRIGGER SOURCE"=1852576, "TRIGGER GLOBAL EXPOSURE"=2049680, "FIRST TRIGGER BEHAVIOR"=2049696, "CHANNEL SYNC"=1852352, "READOUT DIRECTION"=4211904, "PRE HSYNC COUNT"=1852704] ("Parameter")
                n78 = event-data() -> ("NewVal"=w677:sgl)  [unwired: 1 in, 3 out]
                n79 = call <userlib>:"tm_stopcapture.vi"("error in (no error)"=w690, "Handle in"=w687) -> ("error out"=w691:errorcluster, "Handle out"=w686:u32)  [unwired: 8 in]
                n80 = call <userlib>:"tm_unpreparecapture.vi"("error in (no error)"=w691, "Handle in"=w686) -> ("error out"=w689:errorcluster, "Handle out"=w688:u32)  [unwired: 8 in]
                n81 = call <userlib>:"tm_setparameter_a.vi"("error in (no error)"=w689, "Value in"=w677, "Parameter"=w678, "Handle in"=w688) -> ("error out"=w682:errorcluster, "Handle out"=w681:u32)  [unwired: 6 in]
                n82 = call <userlib>:"tm_preparecapture.vi"("error in (no error)"=w682, "Capture mode"=w685, "Handle in"=w681) -> ("error out"=w683:errorcluster, "Handle out"=w684:u32)  [unwired: 5 in, 2 out]
                n83 = call <userlib>:"tm_startcapture_b.vi"("error in (no error)"=w683, "Handle in"=w684) -> ("error out"=w679:errorcluster, "Handle out"=w680:u32)  [unwired: 8 in]
              }
              event "Camera Readout Mode", "Slit Width / Lines": Value Change {
                w702 = 1 items=["Snap", "Sequence"] ("Capture mode")
                n84 = event-data() -> ()  [unwired: 1 in, 4 out]
                n85 = call <userlib>:"tm_stopcapture.vi"("error in (no error)"=w708, "Handle in"=w709) -> ("error out"=w710:errorcluster, "Handle out"=w706:u32)  [unwired: 8 in]
                n86 = call <userlib>:"tm_unpreparecapture.vi"("error in (no error)"=w710, "Handle in"=w706) -> ("error out"=w701:errorcluster, "Handle out"=w707:u32)  [unwired: 8 in]
                n87 = call <userlib>:"tm_setpropertyvalue.vi"("error in (no error)"=w701, "Value in"="Camera Readout Mode", "Property ID"=u32 4194832, "Handle in"=w707) -> ("error out"=w711:errorcluster, "Handle out"=w712:u32)  [unwired: 6 in]
                n88 = case shown="12" "Camera Readout Mode" {
                  tunnel: w712 -> [w723 w730]
                  tunnel: [w722 w725] -> w705
                  tunnel: w711 -> [w720 w735]
                  tunnel: [w719 w735] -> w703
                  frame 1, Default {
                    n89 = local read "Exposure"() -> (w721:dbl)
                    n90 = call <userlib>:"tm_setpropertyvalue.vi"("error in (no error)"=w720, "Value in"=w721, "Property ID"=u32 2031888, "Handle in"=w723) -> ("error out"=w719:errorcluster, "Handle out"=w722:u32)  [unwired: 6 in]
                  }
                  frame 12 {
                    n91 = local read "Exposure"() -> (w734:dbl)
                    n92 = local read "SVW"() -> (w732:i32)
                    n93 = formula code="slitExpos=frameInter*LW/(LinesToReadout\n+10+LW);\nlineInter = slitExpos / LW;"("frameInter"=w734, "LW"="Slit Width / Lines", "LinesToReadout"=w732) -> ("slitExpos"=w726:dbl, "lineInter"=w729:dbl)
                    n94 = call <userlib>:"tm_setpropertyvalue.vi"("Value in"=w729, "Property ID"=u32 4208720, "Handle in"=w730) -> ("Handle out"=w728:u32)  [unwired: 7 in, 1 out]
                    n95 = call <userlib>:"tm_setpropertyvalue.vi"("Value in"=w726, "Property ID"=u32 2031888, "Handle in"=w728) -> ("Handle out"=w725:u32)  [unwired: 7 in, 1 out]
                  }
                }
                n96 = call <userlib>:"tm_preparecapture.vi"("error in (no error)"=w703, "Capture mode"=w702, "Handle in"=w705) -> ("error out"=w698:errorcluster, "Buffer Info"=w704:T7, "Handle out"=w700:u32)  [unwired: 5 in, 1 out]
                n97 = call <userlib>:"tm_startcapture_b.vi"("error in (no error)"=w698, "Handle in"=w700) -> ("error out"=w697:errorcluster, "Handle out"=w699:u32)  [unwired: 8 in]
              }
              event "Ram Record": Value Change {
                n98 = event-data() -> ()  [unwired: 1 in, 5 out]
                n99 = case shown="True" "Ram Record" {
                  tunnel: w749 -> [w753 w776]
                  tunnel: w748 -> [w752 w773]
                  tunnel: [w753 w759] -> w747
                  tunnel: [w752 w761] -> w746
                  tunnel: [w751 w760] -> w742
                  tunnel: w741 -> [w751 _]
                  tunnel: w739 -> [_ w764]
                  tunnel: [_ w762] -> w738
                  tunnel: w737 -> [_ w758]
                  tunnel: w736 -> [_ w754]
                  frame False {
                  }
                  frame True {
                    w770 = 0 items=["Snap", "Sequence"] ("Capture mode")
                    # "Max 2500"
                    n100 = Flush Queue(queue=w764) -> (queue out=w763:refnum<queue>)  [unwired: 1 in, 2 out]
                    n101 = call <userlib>:"tm_stopcapture.vi"("error in (no error)"=w776, "Handle in"=w773) -> ("error out"=w775:errorcluster, "Handle out"=w774:u32)  [unwired: 8 in]
                    n102 = Bundle By Name(cluster=w754, "State"=Stack_Track."Start Sequence", "Stack Number"=0, "Image"=w758) -> (w755:T3)
                    n103 = call <userlib>:"tm_unpreparecapture.vi"("error in (no error)"=w775, "Handle in"=w774) -> ("error out"=w771:errorcluster, "Handle out"=w772:u32)  [unwired: 8 in]
                    n104 = call <userlib>:"tm_preparecapture.vi"("error in (no error)"=w771, "Frames"="Frames", "Capture mode"=w770, "Handle in"=w772) -> ("error out"=w769:errorcluster, "Buffer Info"=w767:T7, "Handle out"=w768:u32)  [unwired: 4 in, 1 out]
                    n105 = Enqueue Element(queue=w763, element=w755) -> (queue out=w765:refnum<queue>)  [unwired: 2 in, 2 out]
                    n106 = case shown="No Error" w769 {
                      selector: w769 -> [w801 w822]
                      tunnel: w768 -> [w800 w823]
                      tunnel: "Frames" -> [w796 _]
                      tunnel: [w781 w819] -> w761
                      tunnel: w767 -> [w797 _]
                      tunnel: [w780 w821] -> w759
                      tunnel: w765 -> [w795 w817]
                      tunnel: w754 -> [w794 _]
                      tunnel: [w779 w817] -> _
                      tunnel: [FALSE ("value") w831] -> w762
                      tunnel: [w778 w820] -> w760
                      frame No Error {
                        w786 = 1 items=["Snap", "Sequence"] ("Capture mode")
                        # "Frames in RAM"
                        n107 = call <userlib>:"tm_startcapture_b.vi"("error in (no error)"=w801, "Handle in"=w800) -> ("error out"=w798:errorcluster, "Handle out"=w799:u32)  [unwired: 8 in]
                        n108 = for {
                          N: w796 -> [_]
                          tunnel: w799 -> [w816]
                          tunnel: w798 -> [w815]
                          tunnel: w797 -> [w812]
                          tunnel: [w811] -> w792
                          tunnel: [w810] -> w791
                          tunnel: w795 -> [w808]
                          tunnel: Stack_Track."Collecting" ("Enum") -> [w806]
                          tunnel: w794 -> [w804]
                          tunnel: [w803] -> w785
                          i -> [w805]
                          n109 = call <userlib>:"tm_waitnextframe.vi"("error in (no error)"=w815, "Handle in"=w816) -> ("error out"=w813:errorcluster, "Frame Index"=→"Frame Index":i32, "Handle out"=w814:u32)  [unwired: 6 in, 1 out]
                          n110 = call <userlib>:"tm_getframe_a.vi"("error in (no error)"=w813, "Frame Index"=w805, "Buffer Info"=w812, "Handle in"=w814) -> ("error out"=w810:errorcluster, "Data 16"=w802:u16[][], "Handle out"=w811:u32)  [unwired: 3 in, 2 out]
                          n111 = Bundle By Name(cluster=w804, "State"=w806, "Stack Number"=w805, "Image"=w802) -> (w807:T3)
                          n112 = Enqueue Element(queue=w808, element=w807) -> (queue out=w803:refnum<queue>)  [unwired: 2 in, 2 out]
                        }
                        n113 = call <userlib>:"tm_stopcapture.vi"("error in (no error)"=w791, "Handle in"=w792) -> ("error out"=w789:errorcluster, "Handle out"=w790:u32)  [unwired: 8 in]
                        n114 = call <userlib>:"tm_unpreparecapture.vi"("error in (no error)"=w789, "Handle in"=w790) -> ("error out"=w788:errorcluster, "Handle out"=w787:u32)  [unwired: 8 in]
                        n115 = Enqueue Element(queue=w785, element=T3 {"State"=enum."End", "Stack Number"=0, "Image"=[], "Stacks"=0} ("input cluster")) -> (queue out=w779:refnum<queue>)  [unwired: 2 in, 2 out]
                        n116 = call <userlib>:"tm_preparecapture.vi"("error in (no error)"=w788, "Capture mode"=w786, "Handle in"=w787) -> ("error out"=w783:errorcluster, "Buffer Info"=w778:T7, "Handle out"=w782:u32)  [unwired: 5 in, 1 out]
                        n117 = call <userlib>:"tm_startcapture_b.vi"("error in (no error)"=w783, "Handle in"=w782) -> ("error out"=w780:errorcluster, "Handle out"=w781:u32)  [unwired: 8 in]
                      }
                      frame Error {
                        w826 = 1 items=["Snap", "Sequence"] ("Capture mode")
                        # "Prepare camera failure, likely too many frames in stack"
                        n118 = One Button Dialog(message="Too many frames in stack", button name ("OK")="OK") -> (true=w831:bool)
                        n119 = call <userlib>:"tm_stopcapture.vi"("error in (no error)"=w822, "Handle in"=w823) -> ("error out"=w829:errorcluster, "Handle out"=w830:u32)  [unwired: 8 in]
                        n120 = call <userlib>:"tm_unpreparecapture.vi"("error in (no error)"=w829, "Handle in"=w830) -> ("error out"=w828:errorcluster, "Handle out"=w827:u32)  [unwired: 8 in]
                        n121 = Enqueue Element(queue=w817, element=T3 {"State"=enum."Idle", "Stack Number"=0, "Image"=[], "Stacks"=0} ("input cluster")) -> ()  [unwired: 2 in, 3 out]
                        n122 = call <userlib>:"tm_preparecapture.vi"("error in (no error)"=w828, "Capture mode"=w826, "Handle in"=w827) -> ("error out"=w825:errorcluster, "Buffer Info"=w820:T7, "Handle out"=w824:u32)  [unwired: 5 in, 1 out]
                        n123 = call <userlib>:"tm_startcapture_b.vi"("error in (no error)"=w825, "Handle in"=w824) -> ("error out"=w821:errorcluster, "Handle out"=w819:u32)  [unwired: 8 in]
                      }
                    }
                  }
                }
              }
              event "HardDisk Record": Value Change {
                n124 = event-data() -> ()  [unwired: 1 in, 5 out]
                n125 = case shown="True" "HardDisk Record" {
                  tunnel: w846 -> [w849 w865]
                  tunnel: w845 -> [w848 w862]
                  tunnel: [w849 w852] -> w844
                  tunnel: [w848 w854] -> w843
                  tunnel: [w847 w853] -> w839
                  tunnel: w838 -> [w847 _]
                  tunnel: w836 -> [_ w850]
                  tunnel: [_ w855] -> w835
                  frame False {
                  }
                  frame True {
                    w859 = 0 items=["Snap", "Sequence"] ("Capture mode")
                    # "Max 50"
                    n126 = call <userlib>:"tm_stopcapture.vi"("error in (no error)"=w865, "Handle in"=w862) -> ("error out"=w864:errorcluster, "Handle out"=w863:u32)  [unwired: 8 in]
                    n127 = call <userlib>:"tm_unpreparecapture.vi"("error in (no error)"=w864, "Handle in"=w863) -> ("error out"=w860:errorcluster, "Handle out"=w861:u32)  [unwired: 8 in]
                    n128 = call <userlib>:"tm_preparecapture.vi"("error in (no error)"=w860, "Frames"="Frames", "Capture mode"=w859, "Handle in"=w861) -> ("error out"=w858:errorcluster, "Buffer Info"=w856:T7, "Handle out"=w857:u32)  [unwired: 4 in, 1 out]
                    n129 = case shown="No Error" w858 {
                      selector: w858 -> [w890 w903]
                      tunnel: w857 -> [w876 w904]
                      tunnel: [w879 w900] -> w854
                      tunnel: w856 -> [w887 _]
                      tunnel: [w878 w902] -> w852
                      tunnel: [FALSE ("value") w912] -> w855
                      tunnel: [w877 w901] -> w853
                      tunnel: "Frames" -> [w873 _]
                      tunnel: w850 -> [w867 w898]
                      frame No Error {
                        w882 = 1 items=["Snap", "Sequence"] ("Capture mode")
                        n130 = call <userlib>:"tm_startrecorder.vi"("frames"=w873, "File"="Temp", "Handle in"=w876) -> ("Handle out"=w875:u32)  [unwired: 7 in, 1 out]
                        n131 = call <userlib>:"tm_startcapture_b.vi"("error in (no error)"=w890, "Handle in"=w875) -> ("error out"=w888:errorcluster, "Handle out"=w889:u32)  [unwired: 8 in]
                        n132 = while {
                          tunnel: w889 -> [w896]
                          tunnel: w888 -> [w895]
                          tunnel: w887 -> [_]
                          tunnel: [w897] -> w885
                          tunnel: w873 -> [w892]
                          stop <- w893 stop-if-true
                          n133 = Wait (ms)(milliseconds to wait=u32 50) -> ()  [unwired: 1 out]
                          n134 = call <userlib>:"tm_getrecorderstatus.vi"("error in (no error)"=w895, "Handle"=w896) -> ("error out"=w897:errorcluster, "Count"=w891:i32)  [unwired: 6 in, 2 out]
                          n135 = Equal?(x=w891, y=w892) -> (x = y?=w893:bool)
                        }
                        n136 = call <userlib>:"tm_stopcapture.vi"("error in (no error)"=w885) -> ("error out"=w872:errorcluster, "Handle out"=w871:u32)  [unwired: 9 in]
                        n137 = call <userlib>:"tm_stoprecorder.vi"("error in (no error)"=w872, "Handle in"=w871) -> ("error out"=w869:errorcluster, "Handle out"=w870:u32)  [unwired: 8 in]
                        n138 = Enqueue Element(queue=w867, element=T3 {"State"=enum."Read Disk", "Stack Number"=0, "Image"=[], "Stacks"=0}, error in (no error)=w869) -> (error out=w868:errorcluster)  [unwired: 1 in, 2 out]
                        n139 = call <userlib>:"tm_unpreparecapture.vi"("error in (no error)"=w868, "Handle in"=w870) -> ("error out"=w884:errorcluster, "Handle out"=w883:u32)  [unwired: 8 in]
                        n140 = call <userlib>:"tm_preparecapture.vi"("error in (no error)"=w884, "Capture mode"=w882, "Handle in"=w883) -> ("error out"=w881:errorcluster, "Buffer Info"=w877:T7, "Handle out"=w880:u32)  [unwired: 5 in, 1 out]
                        n141 = call <userlib>:"tm_startcapture_b.vi"("error in (no error)"=w881, "Handle in"=w880) -> ("error out"=w878:errorcluster, "Handle out"=w879:u32)  [unwired: 8 in]
                      }
                      frame Error {
                        w907 = 1 items=["Snap", "Sequence"] ("Capture mode")
                        # "Prepare camera failure, likely too many frames in stack"
                        n142 = One Button Dialog(message="Too many frames in stack", button name ("OK")="OK") -> (true=w912:bool)
                        n143 = call <userlib>:"tm_stopcapture.vi"("error in (no error)"=w903, "Handle in"=w904) -> ("error out"=w910:errorcluster, "Handle out"=w911:u32)  [unwired: 8 in]
                        n144 = call <userlib>:"tm_unpreparecapture.vi"("error in (no error)"=w910, "Handle in"=w911) -> ("error out"=w909:errorcluster, "Handle out"=w908:u32)  [unwired: 8 in]
                        n145 = Enqueue Element(queue=w898, element=T3 {"State"=enum."STOP", "Stack Number"=0, "Image"=[], "Stacks"=0} ("input cluster")) -> ()  [unwired: 2 in, 3 out]
                        n146 = call <userlib>:"tm_preparecapture.vi"("error in (no error)"=w909, "Capture mode"=w907, "Handle in"=w908) -> ("error out"=w906:errorcluster, "Buffer Info"=w901:T7, "Handle out"=w905:u32)  [unwired: 5 in, 1 out]
                        n147 = call <userlib>:"tm_startcapture_b.vi"("error in (no error)"=w906, "Handle in"=w905) -> ("error out"=w902:errorcluster, "Handle out"=w900:u32)  [unwired: 8 in]
                      }
                    }
                  }
                }
              }
              event "Scan Mode": Value Change {
                w915 = u32 4211872 items=["SENSOR MODE"=4212128, "CCD MODE"=4212384, "READOUT MODE"=4211872, "ACTIVE VIEW INDEX"=4343136, "BITS PER CHANNEL"=4342976, "IMAGE PIXEL TYPE"=4343296, "BINNING"=4215968, "EXPOSURE TIME"=2049184, "CONTRAST GAIN"=3163312, "CONTRAST OFFSET"=3163328, "LIGHT MODE"=2114720, "SENSITIVITY"=2114992, "PHOTON IMAGING MODE"=2115200, "HIGH DYNAMIC RANGE MODE"=3163360, "WHITE BALANCE"=3163568, "TEMPERATURE"=2115232, "TEMPERATURE TARGET"=2115264, "SENSOR COOLER FAN"=2115296, "LINEBUNDLE HEIGHT"=4212192, "MECHANICAL SHUTTER"=2115488, "BACK FOCUS POSITION"=8422304, "TRIGGER CONNECTOR"=1066432, "TRIGGER SOURCE"=1066144, "OUTPUT TRIGGER SOURCE"=1852576, "TRIGGER GLOBAL EXPOSURE"=2049680, "FIRST TRIGGER BEHAVIOR"=2049696, "CHANNEL SYNC"=1852352, "READOUT DIRECTION"=4211904, "PRE HSYNC COUNT"=1852704] ("Parameter")
                w930 = 1 items=["Snap", "Sequence"] ("Capture mode")
                n148 = event-data() -> ("NewVal"=w920:dbl)  [unwired: 1 in, 2 out]
                n149 = call <userlib>:"tm_stopcapture.vi"("error in (no error)"=w931, "Handle in"=w932) -> ("error out"=w933:errorcluster, "Handle out"=w934:u32)  [unwired: 8 in]
                n150 = call <userlib>:"tm_unpreparecapture.vi"("error in (no error)"=w933, "Handle in"=w934) -> ("error out"=w918:errorcluster, "Handle out"=w919:u32)  [unwired: 8 in]
                n151 = call <userlib>:"tm_setparameter_a.vi"("error in (no error)"=w918, "Value in"=w920, "Parameter"=w915, "Handle in"=w919) -> ("error out"=w917:errorcluster, "Handle out"=w916:u32)  [unwired: 6 in]
                n152 = call <userlib>:"tm_getparameter_a.vi"("error in (no error)"=w917, "Parameter"=w915, "Handle in"=w916) -> ("error out"=w923:errorcluster, "Value out"=w922:dbl, "Handle out"=w921:u32)  [unwired: 6 in]
                n153 = local write "SMD"(w922) -> ()
                n154 = call <userlib>:"tm_preparecapture.vi"("error in (no error)"=w923, "Capture mode"=w930, "Handle in"=w921) -> ("error out"=w928:errorcluster, "Buffer Info"=w925:T7, "Handle out"=w929:u32)  [unwired: 5 in, 1 out]
                n155 = call <userlib>:"tm_startcapture_b.vi"("error in (no error)"=w928, "Handle in"=w929) -> ("error out"=w927:errorcluster, "Handle out"=w926:u32)  [unwired: 8 in]
              }
              event "Binning": Value Change {
                w939 = u32 4215968 items=["BINNING"=4215968, "BITS PER CHANNEL"=2, "ACTIVE VIEW INDEX"=3, "CCD MODE"=4, "SENSOR MODE"=5, "READOUT MODE"=6, "EXPOSURE TIME"=7, "CONTRAST GAIN"=8, "CONTRAST OFFSET"=9, "LIGHT MODE"=10, "SENSITIVITY"=11, "WHITE BALANCE"=12, "PHOTON IMAGING MODE"=13, "HIGH DYNAMIC RANGE MODE"=14, "TRIGGER SOURCE"=15, "TRIGGER ACTIVE"=16, "TRIGGER MODE"=17, "TRIGGER POLARITY"=18, "TRIGGER GLOBAL EXPOSURE"=19, "FIRST TRIGGER BEHAVIOR"=20, "TRIGGER TIMES"=21, "OUTPUT TRIGGER POLARITY"=22, "OUTPUT TRIGGER DELAY"=23, "OUTPUT TRIGGER PERIOD"=24, "TEMPERATURE"=25, "TEMPERATURE TARGET"=26, "SENSOR COOLER FAN"=27, "MECHANICAL SHUTTER"=28, "BACK FOCUS POSITION"=29, "FRAMEBUNDLE MODE"=30, "FRAMEBUNDLE NUMBER"=31, "LINEBUNDLE HEIGHT"=32, "TRIGGER CONNECTOR"=33, "IMAGE PIXEL TYPE"=34, "OUTPUT TRIGGER KIND"=35, "READOUT DIRECTION"=36, "CHANNEL SYNC"=37] ("Parameter")
                w978 = 1 items=["Snap", "Sequence"] ("Capture mode")
                n156 = event-data() -> ("NewVal"=w940:u16)  [unwired: 1 in, 2 out]
                n157 = call <userlib>:"tm_stopcapture.vi"("error in (no error)"=w947, "Handle in"=w948) -> ("error out"=w945:errorcluster, "Handle out"=w946:u32)  [unwired: 8 in]
                n158 = call <userlib>:"tm_unpreparecapture.vi"("error in (no error)"=w945, "Handle in"=w946) -> ("error out"=w941:errorcluster, "Handle out"=w938:u32)  [unwired: 8 in]
                n159 = call <userlib>:"tm_setparameter_a.vi"("error in (no error)"=w941, "Value in"=w940, "Parameter"=w939, "Handle in"=w938) -> ("error out"=w942:errorcluster, "Handle out"=w943:u32)  [unwired: 6 in]
                n160 = call <userlib>:"tm_getarea_a.vi"("error in (no error)"=w942, "Handle in"=w943) -> ("error out"=w966:errorcluster, "V Offset"=w968:T6, "H Offset"=w967:T6, "Handle out"=w965:u32, "H Width"=w969:T6, "V Width"=w970:T6)  [unwired: 4 in]
                n161 = Unbundle By Name(w967) -> ("Value"=w961:i32, "Minimum"=w964:i32, "Maximum"=w963:i32, "Increment"=w962:i32)
                n162 = Unbundle By Name(w968) -> ("Value"=w951:i32, "Minimum"=w960:i32, "Maximum"=w959:i32, "Increment"=w958:i32)
                n163 = Unbundle By Name(w969) -> ("Value"=w950:i32, "Minimum"=w957:i32, "Maximum"=w956:i32, "Increment"=w955:i32)
                n164 = Unbundle By Name(w970) -> ("Value"=w949:i32, "Minimum"=w954:i32, "Maximum"=w953:i32, "Increment"=w952:i32)
                n165 = property on="H Offset" class="DigNum (strict)"("Value"=w961, "Minimum"=w964, "Maximum"=w963, "Increment"=w962) -> ()  [unwired: 2 in, 2 out]
                n166 = property on="V Offset" class="DigNum (strict)"("Value"=w951, "Minimum"=w960, "Maximum"=w959, "Increment"=w958) -> ()  [unwired: 2 in, 2 out]
                n167 = property on="H Width" class="DigNum (strict)"("Value"=w950, "Minimum"=w957, "Maximum"=w956, "Increment"=w955) -> ()  [unwired: 2 in, 2 out]
                n168 = property on="V Width" class="DigNum (strict)"("Value"=w949, "Minimum"=w954, "Maximum"=w953, "Increment"=w952) -> ()  [unwired: 2 in, 2 out]
                n169 = local write "SHO"(w961) -> ()
                n170 = local write "SVO"(w951) -> ()
                n171 = local write "SHW"(w950) -> ()
                n172 = local write "SVW"(w949) -> ()
                n173 = call <userlib>:"tm_preparecapture.vi"("error in (no error)"=w966, "Capture mode"=w978, "Handle in"=w965) -> ("error out"=w976:errorcluster, "Buffer Info"=w973:T7, "Handle out"=w977:u32)  [unwired: 5 in, 1 out]
                n174 = call <userlib>:"tm_startcapture_b.vi"("error in (no error)"=w976, "Handle in"=w977) -> ("error out"=w975:errorcluster, "Handle out"=w974:u32)  [unwired: 8 in]
              }
              event "H Offset", "H Width", "V Offset", "V Width": Value Change {
                w1023 = 1 items=["Snap", "Sequence"] ("Capture mode")
                n175 = event-data() -> ()  [unwired: 1 in, 4 out]
                n176 = call <userlib>:"tm_stopcapture.vi"("error in (no error)"=w985, "Handle in"=w986) -> ("error out"=w983:errorcluster, "Handle out"=w984:u32)  [unwired: 8 in]
                n177 = local read "H Offset"() -> (w989:i32)
                n178 = local read "H Width"() -> (w990:i32)
                n179 = local read "V Offset"() -> (w991:i32)
                n180 = local read "V Width"() -> (w988:i32)
                n181 = call <userlib>:"tm_unpreparecapture.vi"("error in (no error)"=w983, "Handle in"=w984) -> ("error out"=w981:errorcluster, "Handle out"=w982:u32)  [unwired: 8 in]
                n182 = Bundle("H Offset"=w989, "V Offset"=w991, "H Width"=w990, "V Width"=w988) -> (w987:T8)  [unwired: 1 in]
                n183 = call <userlib>:"tm_setarea.vi"("error in (no error)"=w981, "Sub Region"=w987, "Handle in"=w982) -> ("error out"=w992:errorcluster, "Handle out"=w993:u32)  [unwired: 7 in]
                n184 = call <userlib>:"tm_getarea_a.vi"("error in (no error)"=w992, "Handle in"=w993) -> ("error out"=w1011:errorcluster, "V Offset"=w1013:T6, "H Offset"=w1012:T6, "Handle out"=w1010:u32, "H Width"=w1014:T6, "V Width"=w1015:T6)  [unwired: 4 in]
                n185 = Unbundle By Name(w1012) -> ("Value"=w1006:i32, "Minimum"=w1009:i32, "Maximum"=w1008:i32, "Increment"=w1007:i32)
                n186 = Unbundle By Name(w1013) -> ("Value"=w996:i32, "Minimum"=w1005:i32, "Maximum"=w1004:i32, "Increment"=w1003:i32)
                n187 = Unbundle By Name(w1014) -> ("Value"=w995:i32, "Minimum"=w1002:i32, "Maximum"=w1001:i32, "Increment"=w1000:i32)
                n188 = Unbundle By Name(w1015) -> ("Value"=w994:i32, "Minimum"=w999:i32, "Maximum"=w998:i32, "Increment"=w997:i32)
                n189 = property on="H Offset" class="DigNum (strict)"("Value"=w1006, "Minimum"=w1009, "Maximum"=w1008, "Increment"=w1007) -> ()  [unwired: 2 in, 2 out]
                n190 = property on="V Offset" class="DigNum (strict)"("Value"=w996, "Minimum"=w1005, "Maximum"=w1004, "Increment"=w1003) -> ()  [unwired: 2 in, 2 out]
                n191 = property on="H Width" class="DigNum (strict)"("Value"=w995, "Minimum"=w1002, "Maximum"=w1001, "Increment"=w1000) -> ()  [unwired: 2 in, 2 out]
                n192 = property on="V Width" class="DigNum (strict)"("Value"=w994, "Minimum"=w999, "Maximum"=w998, "Increment"=w997) -> ()  [unwired: 2 in, 2 out]
                n193 = local write "SHO"(w1006) -> ()
                n194 = local write "SVO"(w996) -> ()
                n195 = local write "SHW"(w995) -> ()
                n196 = local write "SVW"(w994) -> ()
                n197 = call <userlib>:"tm_preparecapture.vi"("error in (no error)"=w1011, "Capture mode"=w1023, "Handle in"=w1010) -> ("error out"=w1021:errorcluster, "Buffer Info"=w1018:T7, "Handle out"=w1022:u32)  [unwired: 5 in, 1 out]
                n198 = call <userlib>:"tm_startcapture_b.vi"("error in (no error)"=w1021, "Handle in"=w1022) -> ("error out"=w1020:errorcluster, "Handle out"=w1019:u32)  [unwired: 8 in]
              }
            }
            n199 = local read "stop"() -> (w527:bool)
            n200 = Unbundle By Name(w536) -> ("status"=w549:bool)
            n201 = Compound Arithmetic op=OR(w549, w527, w531) -> (w548:bool)
          }
        }
        frame Enabled {
        }
      }
      n202 = while {
        tunnel: w9 -> [w130]
        tunnel: w10 -> [w133]
        tunnel: w15 -> [w129]
        shift-right: [w128] -> _
        shift-left: w14 -> [w131]
        shift-right: [w127] -> w8
        shift-left: w13 -> [w132]
        tunnel: w12 -> [w126]
        tunnel: [w120] -> w7
        shift-right: [w118] -> _
        shift-left: _ -> [w117]
        stop <- w119 stop-if-true
        n203 = Dequeue Element(queue=w133, timeout in ms (-1)=1) -> (element=w122:T2, timed out?=w124:bool)  [unwired: 1 in, 2 out]
        n204 = case shown="True" w124 {
          tunnel: [w134 CameraControlTypeDef."Idle" ("Enum")] -> w123
          tunnel: w122 -> [w134 _]
          frame False {
          }
          frame True {
          }
        }
        n205 = case shown="\"Idle\", Default" w123 {
          tunnel: w132 -> [w156 w237 w289 w331 w370 w407 w440 w469 w478 w511 w514]
          tunnel: w131 -> [_ _ _ _ _ w414 w434 _ _ _ w513]
          tunnel: w130 -> [w158 w238 _ _ _ _ w439 _ _ _ _]
          tunnel: w129 -> [w159 _ _ _ _ _ w438 _ _ _ _]
          tunnel: [w155 w233 w302 w340 w377 w414 w434 w455 w476 w494 w513] -> w128
          tunnel: [w154 w234 w295 w338 w375 w415 w433 w459 w475 w507 w514] -> w127
          tunnel: w126 -> [w157 w236 w327 w366 w385 w406 w431 w472 w477 w501 w515]
          tunnel: [w153 w235 w301 w339 w376 w413 w432 w460 w474 w506 w515] -> w120
          tunnel: [w137 w222 w288 w330 w369 w405 w430 w454 w473 w492 w512] -> w118
          tunnel: w117 -> [w136 w222 w288 w330 w369 w405 w428 w454 w473 w492 w512]
          frame "Ram Record" {
            w148 = 0 items=["Snap", "Sequence"] ("Capture mode")
            # "Max 2500"
            n206 = local read "Stack Frames"() -> (w139:i32)
            n207 = Flush Queue(queue=w158) -> (queue out=w143:refnum<queue>)  [unwired: 1 in, 2 out]
            n208 = call <userlib>:"tm_stopcapture.vi"("error in (no error)"=w157, "Handle in"=w156) -> ("error out"=w152:errorcluster, "Handle out"=w151:u32)  [unwired: 8 in]
            n209 = Bundle By Name(cluster=w159, "State"=Stack_Track."Start Sequence", "Stack Number"=0, "Image"=w136) -> (w140:T3)
            n210 = call <userlib>:"tm_unpreparecapture.vi"("error in (no error)"=w152, "Handle in"=w151) -> ("error out"=w149:errorcluster, "Handle out"=w150:u32)  [unwired: 8 in]
            n211 = call <userlib>:"tm_preparecapture.vi"("error in (no error)"=w149, "Frames"=w139, "Capture mode"=w148, "Handle in"=w150) -> ("error out"=w147:errorcluster, "Buffer Info"=w145:T7, "Handle out"=w146:u32)  [unwired: 4 in, 1 out]
            n212 = Enqueue Element(queue=w143, element=w140) -> (queue out=w144:refnum<queue>)  [unwired: 2 in, 2 out]
            n213 = case shown="No Error" w147 {
              selector: w147 -> [w187 w210]
              tunnel: w146 -> [w186 w211]
              tunnel: w139 -> [w182 _]
              tunnel: [w167 w207] -> w154
              tunnel: w145 -> [w183 _]
              tunnel: [w166 w209] -> w153
              tunnel: w144 -> [w181 w205]
              tunnel: w159 -> [w180 _]
              tunnel: [w165 w205] -> _
              tunnel: [FALSE ("value") w219] -> _
              tunnel: [w164 w208] -> w155
              tunnel: [FALSE ("Boolean") _] -> w138
              tunnel: [w161 w204] -> w137
              tunnel: w136 -> [_ w204]
              frame No Error {
                w172 = 1 items=["Snap", "Sequence"] ("Capture mode")
                # "Frames in RAM"
                n214 = call <userlib>:"tm_startcapture_b.vi"("error in (no error)"=w187, "Handle in"=w186) -> ("error out"=w184:errorcluster, "Handle out"=w185:u32)  [unwired: 8 in]
                n215 = for {
                  N: w182 -> [_]
                  tunnel: w185 -> [w203]
                  tunnel: w184 -> [w202]
                  tunnel: w183 -> [w199]
                  tunnel: [w198] -> w178
                  tunnel: [w197] -> w177
                  tunnel: w181 -> [w196]
                  tunnel: Stack_Track."Collecting" ("Enum") -> [w194]
                  tunnel: w180 -> [w192]
                  tunnel: [w191] -> w171
                  tunnel: [w189] -> w161
                  tunnel: TRUE ("Boolean") -> [w188]
                  i -> [w193]
                  n216 = local write "Record Ready"(w188) -> ()
                  n217 = call <userlib>:"tm_waitnextframe.vi"("error in (no error)"=w202, "Handle in"=w203) -> ("error out"=w200:errorcluster, "Frame Index"=w190:i32, "Handle out"=w201:u32)  [unwired: 6 in, 1 out]
                  n218 = call <userlib>:"tm_getframe_a.vi"("error in (no error)"=w200, "Frame Index"=w193, "Buffer Info"=w199, "Handle in"=w201) -> ("error out"=w197:errorcluster, "Data 16"=w189:u16[][], "Handle out"=w198:u32)  [unwired: 3 in, 2 out]
                  n219 = Bundle By Name(cluster=w192, "State"=w194, "Stack Number"=w193, "Image"=w189) -> (w195:T3)
                  n220 = Enqueue Element(queue=w196, element=w195) -> (queue out=w191:refnum<queue>)  [unwired: 2 in, 2 out]
                  n221 = local write "Stack Frames"(w190) -> ()
                }
                n222 = call <userlib>:"tm_stopcapture.vi"("error in (no error)"=w177, "Handle in"=w178) -> ("error out"=w175:errorcluster, "Handle out"=w176:u32)  [unwired: 8 in]
                n223 = call <userlib>:"tm_unpreparecapture.vi"("error in (no error)"=w175, "Handle in"=w176) -> ("error out"=w174:errorcluster, "Handle out"=w173:u32)  [unwired: 8 in]
                n224 = Enqueue Element(queue=w171, element=T3 {"State"=enum."End", "Stack Number"=0, "Image"=[], "Stacks"=0} ("input cluster")) -> (queue out=w165:refnum<queue>)  [unwired: 2 in, 2 out]
                n225 = call <userlib>:"tm_preparecapture.vi"("error in (no error)"=w174, "Capture mode"=w172, "Handle in"=w173) -> ("error out"=w169:errorcluster, "Buffer Info"=w164:T7, "Handle out"=w168:u32)  [unwired: 5 in, 1 out]
                n226 = call <userlib>:"tm_startcapture_b.vi"("error in (no error)"=w169, "Handle in"=w168) -> ("error out"=w166:errorcluster, "Handle out"=w167:u32)  [unwired: 8 in]
              }
              frame Error {
                w214 = 1 items=["Snap", "Sequence"] ("Capture mode")
                # "Prepare camera failure, likely too many frames in stack"
                n227 = One Button Dialog(message="Too many frames in stack", button name ("OK")="OK") -> (true=w219:bool)
                n228 = call <userlib>:"tm_stopcapture.vi"("error in (no error)"=w210, "Handle in"=w211) -> ("error out"=w217:errorcluster, "Handle out"=w218:u32)  [unwired: 8 in]
                n229 = call <userlib>:"tm_unpreparecapture.vi"("error in (no error)"=w217, "Handle in"=w218) -> ("error out"=w216:errorcluster, "Handle out"=w215:u32)  [unwired: 8 in]
                n230 = Enqueue Element(queue=w205, element=T3 {"State"=enum."Idle", "Stack Number"=0, "Image"=[], "Stacks"=0} ("input cluster")) -> ()  [unwired: 2 in, 3 out]
                n231 = call <userlib>:"tm_preparecapture.vi"("error in (no error)"=w216, "Capture mode"=w214, "Handle in"=w215) -> ("error out"=w213:errorcluster, "Buffer Info"=w208:T7, "Handle out"=w212:u32)  [unwired: 5 in, 1 out]
                n232 = call <userlib>:"tm_startcapture_b.vi"("error in (no error)"=w213, "Handle in"=w212) -> ("error out"=w209:errorcluster, "Handle out"=w207:u32)  [unwired: 8 in]
              }
            }
            n233 = local write "Record Ready"(w138) -> ()
          }
          frame "HardDisk Record" {
            w228 = 0 items=["Snap", "Sequence"] ("Capture mode")
            # "Would add for loop here"
            # "Max 50"
            n234 = local read "Stack Frames"() -> (w224:i32)
            n235 = call <userlib>:"tm_stopcapture.vi"("error in (no error)"=w236, "Handle in"=w237) -> ("error out"=w232:errorcluster, "Handle out"=w231:u32)  [unwired: 8 in]
            n236 = call <userlib>:"tm_unpreparecapture.vi"("error in (no error)"=w232, "Handle in"=w231) -> ("error out"=w229:errorcluster, "Handle out"=w230:u32)  [unwired: 8 in]
            n237 = call <userlib>:"tm_preparecapture.vi"("error in (no error)"=w229, "Frames"=w224, "Capture mode"=w228, "Handle in"=w230) -> ("error out"=w227:errorcluster, "Buffer Info"=w225:T7, "Handle out"=w226:u32)  [unwired: 4 in, 1 out]
            n238 = case shown="No Error" w227 {
              selector: w227 -> [w263 w276]
              tunnel: w226 -> [w249 w277]
              tunnel: [w252 w273] -> w234
              tunnel: w225 -> [w260 _]
              tunnel: [w251 w275] -> w235
              tunnel: [FALSE ("value") w285] -> _
              tunnel: [w250 w274] -> w233
              tunnel: w224 -> [w247 _]
              tunnel: w238 -> [w241 w271]
              tunnel: path "C:/temp.tmp" ("Temp 2") -> [w239 _]
              frame No Error {
                w255 = 1 items=["Snap", "Sequence"] ("Capture mode")
                n239 = call <userlib>:"tm_startrecorder.vi"("frames"=w247, "File"=w239, "Handle in"=w249) -> ("Handle out"=w248:u32)  [unwired: 7 in, 1 out]
                n240 = call <userlib>:"tm_startcapture_b.vi"("error in (no error)"=w263, "Handle in"=w248) -> ("error out"=w261:errorcluster, "Handle out"=w262:u32)  [unwired: 8 in]
                n241 = while {
                  tunnel: w262 -> [w269]
                  tunnel: w261 -> [w268]
                  tunnel: w260 -> [_]
                  tunnel: [w270] -> w258
                  tunnel: w247 -> [w265]
                  stop <- w266 stop-if-true
                  n242 = Wait (ms)(milliseconds to wait=u32 50) -> ()  [unwired: 1 out]
                  n243 = call <userlib>:"tm_getrecorderstatus.vi"("error in (no error)"=w268, "Handle"=w269) -> ("error out"=w270:errorcluster, "Count"=w264:i32)  [unwired: 6 in, 2 out]
                  n244 = Equal?(x=w264, y=w265) -> (x = y?=w266:bool)
                }
                n245 = call <userlib>:"tm_stopcapture.vi"("error in (no error)"=w258) -> ("error out"=w246:errorcluster, "Handle out"=w245:u32)  [unwired: 9 in]
                n246 = call <userlib>:"tm_stoprecorder.vi"("error in (no error)"=w246, "Handle in"=w245) -> ("error out"=w243:errorcluster, "Handle out"=w244:u32)  [unwired: 8 in]
                n247 = Enqueue Element(queue=w241, element=T3 {"State"=enum."Read Disk", "Stack Number"=0, "Image"=[], "Stacks"=0}, error in (no error)=w243) -> (error out=w242:errorcluster)  [unwired: 1 in, 2 out]
                n248 = call <userlib>:"tm_unpreparecapture.vi"("error in (no error)"=w242, "Handle in"=w244) -> ("error out"=w257:errorcluster, "Handle out"=w256:u32)  [unwired: 8 in]
                n249 = call <userlib>:"tm_preparecapture.vi"("error in (no error)"=w257, "Capture mode"=w255, "Handle in"=w256) -> ("error out"=w254:errorcluster, "Buffer Info"=w250:T7, "Handle out"=w253:u32)  [unwired: 5 in, 1 out]
                n250 = call <userlib>:"tm_startcapture_b.vi"("error in (no error)"=w254, "Handle in"=w253) -> ("error out"=w251:errorcluster, "Handle out"=w252:u32)  [unwired: 8 in]
              }
              frame Error {
                w280 = 1 items=["Snap", "Sequence"] ("Capture mode")
                # "Prepare camera failure, likely too many frames in stack"
                n251 = One Button Dialog(message="Too many frames in stack", button name ("OK")="OK") -> (true=w285:bool)
                n252 = call <userlib>:"tm_stopcapture.vi"("error in (no error)"=w276, "Handle in"=w277) -> ("error out"=w283:errorcluster, "Handle out"=w284:u32)  [unwired: 8 in]
                n253 = call <userlib>:"tm_unpreparecapture.vi"("error in (no error)"=w283, "Handle in"=w284) -> ("error out"=w282:errorcluster, "Handle out"=w281:u32)  [unwired: 8 in]
                n254 = Enqueue Element(queue=w271, element=T3 {"State"=enum."STOP", "Stack Number"=0, "Image"=[], "Stacks"=0} ("input cluster")) -> ()  [unwired: 2 in, 3 out]
                n255 = call <userlib>:"tm_preparecapture.vi"("error in (no error)"=w282, "Capture mode"=w280, "Handle in"=w281) -> ("error out"=w279:errorcluster, "Buffer Info"=w274:T7, "Handle out"=w278:u32)  [unwired: 5 in, 1 out]
                n256 = call <userlib>:"tm_startcapture_b.vi"("error in (no error)"=w279, "Handle in"=w278) -> ("error out"=w275:errorcluster, "Handle out"=w273:u32)  [unwired: 8 in]
              }
            }
          }
          frame "ROI" {
            w305 = 1 items=["Snap", "Sequence"] ("Capture mode")
            n257 = call <userlib>:"tm_stopcapture.vi"("error in (no error)"=w327, "Handle in"=w289) -> ("error out"=w328:errorcluster, "Handle out"=w329:u32)  [unwired: 8 in]
            n258 = call <userlib>:"tm_unpreparecapture.vi"("error in (no error)"=w328, "Handle in"=w329) -> ("error out"=w291:errorcluster, "Handle out"=w292:u32)  [unwired: 8 in]
            n259 = local read "V Width"() -> (w297:i32)
            n260 = local read "V Offset"() -> (w299:i32)
            n261 = local read "H Width"() -> (w298:i32)
            n262 = local read "H Offset"() -> (w300:i32)
            n263 = Bundle("H Offset"=w300, "V Offset"=w299, "H Width"=w298, "V Width"=w297) -> (w296:T8)  [unwired: 1 in]
            n264 = call <userlib>:"tm_setarea.vi"("error in (no error)"=w291, "Sub Region"=w296, "Handle in"=w292) -> ("error out"=w294:errorcluster, "Handle out"=w293:u32)  [unwired: 7 in]
            n265 = call <userlib>:"tm_getarea_a.vi"("error in (no error)"=w294, "Handle in"=w293) -> ("error out"=w306:errorcluster, "V Offset"=w309:T6, "H Offset"=w310:T6, "Handle out"=w290:u32, "H Width"=w308:T6, "V Width"=w307:T6)  [unwired: 4 in]
            n266 = Unbundle By Name(w310) -> ("Value"=w314:i32, "Minimum"=w311:i32, "Maximum"=w312:i32, "Increment"=w313:i32)
            n267 = Unbundle By Name(w309) -> ("Value"=w324:i32, "Minimum"=w315:i32, "Maximum"=w316:i32, "Increment"=w317:i32)
            n268 = Unbundle By Name(w308) -> ("Value"=w325:i32, "Minimum"=w318:i32, "Maximum"=w319:i32, "Increment"=w320:i32)
            n269 = Unbundle By Name(w307) -> ("Value"=w326:i32, "Minimum"=w321:i32, "Maximum"=w322:i32, "Increment"=w323:i32)
            n270 = property on="H Offset" class="DigNum (strict)"("Value"=w314, "Minimum"=w311, "Maximum"=w312, "Increment"=w313) -> ()  [unwired: 2 in, 2 out]
            n271 = property on="V Offset" class="DigNum (strict)"("Value"=w324, "Minimum"=w315, "Maximum"=w316, "Increment"=w317) -> ()  [unwired: 2 in, 2 out]
            n272 = property on="H Width" class="DigNum (strict)"("Value"=w325, "Minimum"=w318, "Maximum"=w319, "Increment"=w320) -> ()  [unwired: 2 in, 2 out]
            n273 = property on="V Width" class="DigNum (strict)"("Value"=w326, "Minimum"=w321, "Maximum"=w322, "Increment"=w323) -> ()  [unwired: 2 in, 2 out]
            n274 = local write "SHO"(w314) -> ()
            n275 = local write "SVO"(w324) -> ()
            n276 = local write "SHW"(w325) -> ()
            n277 = local write "SVW"(w326) -> ()
            n278 = call <userlib>:"tm_preparecapture.vi"("error in (no error)"=w306, "Capture mode"=w305, "Handle in"=w290) -> ("error out"=w304:errorcluster, "Buffer Info"=w302:T7, "Handle out"=w303:u32)  [unwired: 5 in, 1 out]
            n279 = call <userlib>:"tm_startcapture_b.vi"("error in (no error)"=w304, "Handle in"=w303) -> ("error out"=w301:errorcluster, "Handle out"=w295:u32)  [unwired: 8 in]
          }
          frame "Binning" {
            w343 = 1 items=["Snap", "Sequence"] ("Capture mode")
            w333 = u32 4215968 items=["BINNING"=4215968, "BITS PER CHANNEL"=2, "ACTIVE VIEW INDEX"=3, "CCD MODE"=4, "SENSOR MODE"=5, "READOUT MODE"=6, "EXPOSURE TIME"=7, "CONTRAST GAIN"=8, "CONTRAST OFFSET"=9, "LIGHT MODE"=10, "SENSITIVITY"=11, "WHITE BALANCE"=12, "PHOTON IMAGING MODE"=13, "HIGH DYNAMIC RANGE MODE"=14, "TRIGGER SOURCE"=15, "TRIGGER ACTIVE"=16, "TRIGGER MODE"=17, "TRIGGER POLARITY"=18, "TRIGGER GLOBAL EXPOSURE"=19, "FIRST TRIGGER BEHAVIOR"=20, "TRIGGER TIMES"=21, "OUTPUT TRIGGER POLARITY"=22, "OUTPUT TRIGGER DELAY"=23, "OUTPUT TRIGGER PERIOD"=24, "TEMPERATURE"=25, "TEMPERATURE TARGET"=26, "SENSOR COOLER FAN"=27, "MECHANICAL SHUTTER"=28, "BACK FOCUS POSITION"=29, "FRAMEBUNDLE MODE"=30, "FRAMEBUNDLE NUMBER"=31, "LINEBUNDLE HEIGHT"=32, "TRIGGER CONNECTOR"=33, "IMAGE PIXEL TYPE"=34, "OUTPUT TRIGGER KIND"=35, "READOUT DIRECTION"=36, "CHANNEL SYNC"=37] ("Parameter")
            n280 = local read "Binning"() -> (w365:u16)
            n281 = call <userlib>:"tm_stopcapture.vi"("error in (no error)"=w366, "Handle in"=w331) -> ("error out"=w367:errorcluster, "Handle out"=w368:u32)  [unwired: 8 in]
            n282 = call <userlib>:"tm_unpreparecapture.vi"("error in (no error)"=w367, "Handle in"=w368) -> ("error out"=w336:errorcluster, "Handle out"=w337:u32)  [unwired: 8 in]
            n283 = call <userlib>:"tm_setparameter_a.vi"("error in (no error)"=w336, "Value in"=w365, "Parameter"=w333, "Handle in"=w337) -> ("error out"=w334:errorcluster, "Handle out"=w332:u32)  [unwired: 6 in]
            n284 = call <userlib>:"tm_getarea_a.vi"("error in (no error)"=w334, "Handle in"=w332) -> ("error out"=w344:errorcluster, "V Offset"=w347:T6, "H Offset"=w348:T6, "Handle out"=w335:u32, "H Width"=w346:T6, "V Width"=w345:T6)  [unwired: 4 in]
            n285 = Unbundle By Name(w348) -> ("Value"=w352:i32, "Minimum"=w349:i32, "Maximum"=w350:i32, "Increment"=w351:i32)
            n286 = Unbundle By Name(w347) -> ("Value"=w362:i32, "Minimum"=w353:i32, "Maximum"=w354:i32, "Increment"=w355:i32)
            n287 = Unbundle By Name(w346) -> ("Value"=w363:i32, "Minimum"=w356:i32, "Maximum"=w357:i32, "Increment"=w358:i32)
            n288 = Unbundle By Name(w345) -> ("Value"=w364:i32, "Minimum"=w359:i32, "Maximum"=w360:i32, "Increment"=w361:i32)
            n289 = property on="H Offset" class="DigNum (strict)"("Value"=w352, "Minimum"=w349, "Maximum"=w350, "Increment"=w351) -> ()  [unwired: 2 in, 2 out]
            n290 = property on="V Offset" class="DigNum (strict)"("Value"=w362, "Minimum"=w353, "Maximum"=w354, "Increment"=w355) -> ()  [unwired: 2 in, 2 out]
            n291 = property on="H Width" class="DigNum (strict)"("Value"=w363, "Minimum"=w356, "Maximum"=w357, "Increment"=w358) -> ()  [unwired: 2 in, 2 out]
            n292 = property on="V Width" class="DigNum (strict)"("Value"=w364, "Minimum"=w359, "Maximum"=w360, "Increment"=w361) -> ()  [unwired: 2 in, 2 out]
            n293 = local write "SHO"(w352) -> ()
            n294 = local write "SVO"(w362) -> ()
            n295 = local write "SHW"(w363) -> ()
            n296 = local write "SVW"(w364) -> ()
            n297 = call <userlib>:"tm_preparecapture.vi"("error in (no error)"=w344, "Capture mode"=w343, "Handle in"=w335) -> ("error out"=w342:errorcluster, "Buffer Info"=w340:T7, "Handle out"=w341:u32)  [unwired: 5 in, 1 out]
            n298 = call <userlib>:"tm_startcapture_b.vi"("error in (no error)"=w342, "Handle in"=w341) -> ("error out"=w339:errorcluster, "Handle out"=w338:u32)  [unwired: 8 in]
          }
          frame "Readout Mode" {
            w380 = 1 items=["Snap", "Sequence"] ("Capture mode")
            n299 = call <userlib>:"tm_stopcapture.vi"("error in (no error)"=w385, "Handle in"=w370) -> ("error out"=w386:errorcluster, "Handle out"=w387:u32)  [unwired: 8 in]
            n300 = call <userlib>:"tm_unpreparecapture.vi"("error in (no error)"=w386, "Handle in"=w387) -> ("error out"=w371:errorcluster, "Handle out"=w372:u32)  [unwired: 8 in]
            n301 = local read "Camera Readout Mode"() -> (w383:u16)
            n302 = call <userlib>:"tm_setpropertyvalue.vi"("error in (no error)"=w371, "Value in"=w383, "Property ID"=u32 4194832, "Handle in"=w372) -> ("error out"=w381:errorcluster, "Handle out"=w382:u32)  [unwired: 6 in]
            n303 = case shown="12" w383 {
              tunnel: [w391 w396] -> w374
              tunnel: w382 -> [w390 w397]
              tunnel: w381 -> [w389 w396]
              tunnel: [w388 w395] -> w373
              frame 1, Default {
                n304 = local read "Exposure"() -> (w392:dbl)
                n305 = call <userlib>:"tm_setpropertyvalue.vi"("error in (no error)"=w389, "Value in"=w392, "Property ID"=u32 2031888, "Handle in"=w390) -> ("error out"=w391:errorcluster, "Handle out"=w388:u32)  [unwired: 6 in]
              }
              frame 12 {
                n306 = local read "Slit Width / Lines"() -> (w394:sgl)
                n307 = local read "Exposure"() -> (w404:dbl)
                n308 = local read "SVW"() -> (w403:i32)
                n309 = formula code="slitExpos=frameInter*LW/(LinesToReadout\n+10+LW);\nlineInter = slitExpos / LW;"("frameInter"=w404, "LW"=w394, "LinesToReadout"=w403) -> ("slitExpos"=w398:dbl, "lineInter"=w401:dbl)
                n310 = call <userlib>:"tm_setpropertyvalue.vi"("Value in"=w401, "Property ID"=u32 4208720, "Handle in"=w397) -> ("Handle out"=w400:u32)  [unwired: 7 in, 1 out]
                n311 = call <userlib>:"tm_setpropertyvalue.vi"("Value in"=w398, "Property ID"=u32 2031888, "Handle in"=w400) -> ("Handle out"=w395:u32)  [unwired: 7 in, 1 out]
              }
            }
            n312 = call <userlib>:"tm_preparecapture.vi"("error in (no error)"=w374, "Capture mode"=w380, "Handle in"=w373) -> ("error out"=w379:errorcluster, "Buffer Info"=w377:T7, "Handle out"=w378:u32)  [unwired: 5 in, 1 out]
            n313 = call <userlib>:"tm_startcapture_b.vi"("error in (no error)"=w379, "Handle in"=w378) -> ("error out"=w376:errorcluster, "Handle out"=w375:u32)  [unwired: 8 in]
          }
          frame "Update" {
            w411 = u32 1066144 items=["SENSOR MODE"=4212128, "CCD MODE"=4212384, "READOUT MODE"=4211872, "ACTIVE VIEW INDEX"=4343136, "BITS PER CHANNEL"=4342976, "IMAGE PIXEL TYPE"=4343296, "BINNING"=4215968, "EXPOSURE TIME"=2049184, "CONTRAST GAIN"=3163312, "CONTRAST OFFSET"=3163328, "LIGHT MODE"=2114720, "SENSITIVITY"=2114992, "PHOTON IMAGING MODE"=2115200, "HIGH DYNAMIC RANGE MODE"=3163360, "WHITE BALANCE"=3163568, "TEMPERATURE"=2115232, "TEMPERATURE TARGET"=2115264, "SENSOR COOLER FAN"=2115296, "LINEBUNDLE HEIGHT"=4212192, "MECHANICAL SHUTTER"=2115488, "BACK FOCUS POSITION"=8422304, "TRIGGER CONNECTOR"=1066432, "TRIGGER SOURCE"=1066144, "OUTPUT TRIGGER SOURCE"=1852576, "TRIGGER GLOBAL EXPOSURE"=2049680, "FIRST TRIGGER BEHAVIOR"=2049696, "CHANNEL SYNC"=1852352, "READOUT DIRECTION"=4211904, "PRE HSYNC COUNT"=1852704] ("Parameter")
            w416 = u32 2049184 items=["SENSOR MODE"=4212128, "CCD MODE"=4212384, "READOUT MODE"=4211872, "ACTIVE VIEW INDEX"=4343136, "BITS PER CHANNEL"=4342976, "IMAGE PIXEL TYPE"=4343296, "BINNING"=4215968, "EXPOSURE TIME"=2049184, "CONTRAST GAIN"=3163312, "CONTRAST OFFSET"=3163328, "LIGHT MODE"=2114720, "SENSITIVITY"=2114992, "PHOTON IMAGING MODE"=2115200, "HIGH DYNAMIC RANGE MODE"=3163360, "WHITE BALANCE"=3163568, "TEMPERATURE"=2115232, "TEMPERATURE TARGET"=2115264, "SENSOR COOLER FAN"=2115296, "LINEBUNDLE HEIGHT"=4212192, "MECHANICAL SHUTTER"=2115488, "BACK FOCUS POSITION"=8422304, "TRIGGER CONNECTOR"=1066432, "TRIGGER SOURCE"=1066144, "OUTPUT TRIGGER SOURCE"=1852576, "TRIGGER GLOBAL EXPOSURE"=2049680, "FIRST TRIGGER BEHAVIOR"=2049696, "CHANNEL SYNC"=1852352, "READOUT DIRECTION"=4211904, "PRE HSYNC COUNT"=1852704] ("Parameter")
            # "Fails"
            # "Error on get"
            n314 = local read "Exposure"() -> (w418:dbl)
            n315 = disable-structure shown="Enabled" {
              disable-tunnel: w407 -> [w422 _]
              disable-tunnel: w406 -> [w421 _]
              frame Disabled {
                w427 = u32 4191424 items=["SENSOR MODE"=4212128, "CCD MODE"=4212384, "READOUT MODE"=4211872, "ACTIVE VIEW INDEX"=4343136, "BITS PER CHANNEL"=4342976, "IMAGE PIXEL TYPE"=4343296, "BINNING"=4215968, "EXPOSURE TIME"=2049184, "CONTRAST GAIN"=3163312, "CONTRAST OFFSET"=3163328, "LIGHT MODE"=2114720, "SENSITIVITY"=2114992, "PHOTON IMAGING MODE"=2115200, "HIGH DYNAMIC RANGE MODE"=3163360, "WHITE BALANCE"=3163568, "TEMPERATURE"=2115232, "TEMPERATURE TARGET"=2115264, "SENSOR COOLER FAN"=2115296, "LINEBUNDLE HEIGHT"=4212192, "MECHANICAL SHUTTER"=2115488, "BACK FOCUS POSITION"=8422304, "TRIGGER CONNECTOR"=1066432, "TRIGGER SOURCE"=1066144, "OUTPUT TRIGGER SOURCE"=1852576, "TRIGGER GLOBAL EXPOSURE"=2049680, "FIRST TRIGGER BEHAVIOR"=2049696, "CHANNEL SYNC"=1852352, "READOUT DIRECTION"=4211904, "PRE HSYNC COUNT"=1852704, "INTERNAL LINE SPEED"=4191408, "INTERNAL LINE INVERVAL"=4191424] ("Parameter")
                n316 = local read "Internal Line Interval"() -> (w424:dbl)
                n317 = call <userlib>:"tm_setparameter_a.vi"("error in (no error)"=w421, "Value in"=w424, "Parameter"=w427, "Handle in"=w422) -> ("error out"=w423:errorcluster, "Handle out"=w426:u32)  [unwired: 6 in]
                n318 = call <userlib>:"tm_getparameter_a.vi"("error in (no error)"=w423, "Parameter"=w427, "Handle in"=w426) -> ("Value out"=w425:dbl)  [unwired: 6 in, 2 out]
                n319 = local write "Internal Line Interval"(w425) -> ()
              }
              frame Enabled {
              }
            }
            n320 = call <userlib>:"tm_setparameter_a.vi"("error in (no error)"=w406, "Value in"=w418, "Parameter"=w416, "Handle in"=w407) -> ("error out"=w420:errorcluster, "Handle out"=w417:u32)  [unwired: 6 in]
            n321 = call <userlib>:"tm_getparameter_a.vi"("error in (no error)"=w420, "Parameter"=w416, "Handle in"=w417) -> ("Value out"=w419:dbl)  [unwired: 6 in, 2 out]
            n322 = local write "EXP"(w419) -> ()
            n323 = local read "Trigger Source"() -> (w409:sgl)
            n324 = call <userlib>:"tm_setparameter_a.vi"("error in (no error)"=w406, "Value in"=w409, "Parameter"=w411, "Handle in"=w407) -> ("error out"=w408:errorcluster, "Handle out"=w412:u32)  [unwired: 6 in]
            n325 = call <userlib>:"tm_getparameter_a.vi"("error in (no error)"=w408, "Parameter"=w411, "Handle in"=w412) -> ("error out"=w413:errorcluster, "Value out"=w410:dbl, "Handle out"=w415:u32)  [unwired: 6 in]
            n326 = local write "Trigger Source"(w410) -> ()
          }
          frame "Idle", Default {
            # "Slows it all down somewhat"
            # "Currently the external trigger setting means that frames are dropped because the system lingers at this point. \nIdeally I should set it so when the system is external and recording it won't run this section.\n\nThis is what HC Image does, it offers no live video when you switch from live to record mode.\n\nRealistically when tirgger set external and this times out once then ignore this step.\nBut it'd have to be reset after a recording.\n\nNeed to think more betterer about how to handle this else frames will just be dropped. Probably best to just have a seperate scan mode\nOr at least just a boolean to turn off this live capture section."
            n327 = case shown="True" "Capture Mode" {
              tunnel: w440 -> [w442 w453]
              tunnel: w434 -> [_ w451]
              tunnel: [w442 w450] -> w433
              tunnel: [w444 w449] -> w432
              tunnel: w431 -> [w444 w448]
              tunnel: [w443 w446] -> w430
              tunnel: w428 -> [w443 _]
              frame True {
                n328 = Wait (ms)(milliseconds to wait=u32 40) -> ()  [unwired: 1 out]
              }
              frame False {
                n329 = call <userlib>:"tm_waitnextframe.vi"("error in (no error)"=w448, "Timeout"=3000, "Handle in"=w453) -> ("error out"=w447:errorcluster, "Handle out"=w452:u32)  [unwired: 5 in, 2 out]
                n330 = call <userlib>:"tm_getframe_a.vi"("error in (no error)"=w447, "Buffer Info"=w451, "Handle in"=w452) -> ("error out"=w449:errorcluster, "Data 16"=w446:u16[][], "Handle out"=w450:u32)  [unwired: 4 in, 2 out]
              }
            }
            n331 = Bundle By Name(cluster=w438, "State"=Stack_Track."Idle", "Stack Number"=0, "Image"=w430) -> (w435:T3)
            n332 = Enqueue Element(queue=w439, element=w435) -> ()  [unwired: 2 in, 3 out]
          }
          frame "Scan Mode" {
            w456 = 1 items=["Snap", "Sequence"] ("Capture mode")
            w465 = u32 4211872 items=["SENSOR MODE"=4212128, "CCD MODE"=4212384, "READOUT MODE"=4211872, "ACTIVE VIEW INDEX"=4343136, "BITS PER CHANNEL"=4342976, "IMAGE PIXEL TYPE"=4343296, "BINNING"=4215968, "EXPOSURE TIME"=2049184, "CONTRAST GAIN"=3163312, "CONTRAST OFFSET"=3163328, "LIGHT MODE"=2114720, "SENSITIVITY"=2114992, "PHOTON IMAGING MODE"=2115200, "HIGH DYNAMIC RANGE MODE"=3163360, "WHITE BALANCE"=3163568, "TEMPERATURE"=2115232, "TEMPERATURE TARGET"=2115264, "SENSOR COOLER FAN"=2115296, "LINEBUNDLE HEIGHT"=4212192, "MECHANICAL SHUTTER"=2115488, "BACK FOCUS POSITION"=8422304, "TRIGGER CONNECTOR"=1066432, "TRIGGER SOURCE"=1066144, "OUTPUT TRIGGER SOURCE"=1852576, "TRIGGER GLOBAL EXPOSURE"=2049680, "FIRST TRIGGER BEHAVIOR"=2049696, "CHANNEL SYNC"=1852352, "READOUT DIRECTION"=4211904, "PRE HSYNC COUNT"=1852704] ("Parameter")
            n333 = call <userlib>:"tm_stopcapture.vi"("error in (no error)"=w472, "Handle in"=w469) -> ("error out"=w471:errorcluster, "Handle out"=w470:u32)  [unwired: 8 in]
            n334 = call <userlib>:"tm_unpreparecapture.vi"("error in (no error)"=w471, "Handle in"=w470) -> ("error out"=w467:errorcluster, "Handle out"=w468:u32)  [unwired: 8 in]
            n335 = local read "Scan Mode"() -> (w466:dbl)
            n336 = call <userlib>:"tm_setparameter_a.vi"("error in (no error)"=w467, "Value in"=w466, "Parameter"=w465, "Handle in"=w468) -> ("error out"=w461:errorcluster)  [unwired: 6 in, 1 out]
            n337 = call <userlib>:"tm_getparameter_a.vi"("error in (no error)"=w461, "Parameter"=w465) -> ("error out"=w462:errorcluster, "Value out"=w464:dbl, "Handle out"=w457:u32)  [unwired: 7 in]
            n338 = local write "SMD"(w464) -> ()
            n339 = call <userlib>:"tm_preparecapture.vi"("error in (no error)"=w462, "Capture mode"=w456, "Handle in"=w457) -> ("error out"=w463:errorcluster, "Buffer Info"=w455:T7, "Handle out"=w458:u32)  [unwired: 5 in, 1 out]
            n340 = call <userlib>:"tm_startcapture_b.vi"("error in (no error)"=w463, "Handle in"=w458) -> ("error out"=w460:errorcluster, "Handle out"=w459:u32)  [unwired: 8 in]
          }
          frame "Trigger Mode" {
            w479 = u32 1049104 ("Property ID")
            n341 = local read "Trigger Mode"() -> (w484:sgl)
            n342 = call <userlib>:"tm_stopcapture.vi"("error in (no error)"=w477, "Handle in"=w478) -> ("error out"=w483:errorcluster, "Handle out"=w491:u32)  [unwired: 8 in]
            n343 = call <userlib>:"tm_unpreparecapture.vi"("error in (no error)"=w483, "Handle in"=w491) -> ("error out"=w481:errorcluster, "Handle out"=w487:u32)  [unwired: 8 in]
            n344 = call <userlib>:"tm_setpropertyvalue.vi"("error in (no error)"=w481, "Value in"=w484, "Property ID"=w479, "Handle in"=w487) -> ("error out"=w480:errorcluster, "Handle out"=w486:u32)  [unwired: 6 in]
            n345 = call <userlib>:"tm_getpropertyvalue.vi"("error in (no error)"=w480, "Property ID"=w479, "Handle in"=w486) -> ("error out"=w488:errorcluster, "Value in"=w485:sgl, "Handle out"=w489:u32)  [unwired: 6 in]
            n346 = local write "Trigger Mode"(w485) -> ()
            n347 = call <userlib>:"tm_preparecapture.vi"("error in (no error)"=w488, "Handle in"=w489) -> ("error out"=w482:errorcluster, "Buffer Info"=w476:T7, "Handle out"=w490:u32)  [unwired: 6 in, 1 out]
            n348 = call <userlib>:"tm_startcapture_b.vi"("error in (no error)"=w482, "Handle in"=w490) -> ("error out"=w474:errorcluster, "Handle out"=w475:u32)  [unwired: 8 in]
          }
          frame "Readout Direction" {
            w502 = 1 items=["Snap", "Sequence"] ("Capture mode")
            w496 = u32 4211904 items=["SENSOR MODE"=4212128, "CCD MODE"=4212384, "READOUT MODE"=4211872, "ACTIVE VIEW INDEX"=4343136, "BITS PER CHANNEL"=4342976, "IMAGE PIXEL TYPE"=4343296, "BINNING"=4215968, "EXPOSURE TIME"=2049184, "CONTRAST GAIN"=3163312, "CONTRAST OFFSET"=3163328, "LIGHT MODE"=2114720, "SENSITIVITY"=2114992, "PHOTON IMAGING MODE"=2115200, "HIGH DYNAMIC RANGE MODE"=3163360, "WHITE BALANCE"=3163568, "TEMPERATURE"=2115232, "TEMPERATURE TARGET"=2115264, "SENSOR COOLER FAN"=2115296, "LINEBUNDLE HEIGHT"=4212192, "MECHANICAL SHUTTER"=2115488, "BACK FOCUS POSITION"=8422304, "TRIGGER CONNECTOR"=1066432, "TRIGGER SOURCE"=1066144, "OUTPUT TRIGGER SOURCE"=1852576, "TRIGGER GLOBAL EXPOSURE"=2049680, "FIRST TRIGGER BEHAVIOR"=2049696, "CHANNEL SYNC"=1852352, "READOUT DIRECTION"=4211904, "PRE HSYNC COUNT"=1852704] ("Parameter")
            n349 = call <userlib>:"tm_stopcapture.vi"("error in (no error)"=w501, "Handle in"=w511) -> ("error out"=w503:errorcluster, "Handle out"=w510:u32)  [unwired: 8 in]
            n350 = call <userlib>:"tm_unpreparecapture.vi"("error in (no error)"=w503, "Handle in"=w510) -> ("error out"=w504:errorcluster, "Handle out"=w509:u32)  [unwired: 8 in]
            n351 = local read "Readout Direction"() -> (w493:sgl)
            n352 = call <userlib>:"tm_setparameter_a.vi"("error in (no error)"=w504, "Value in"=w493, "Parameter"=w496, "Handle in"=w509) -> ("error out"=w498:errorcluster, "Handle out"=w500:u32)  [unwired: 6 in]
            n353 = call <userlib>:"tm_getparameter_a.vi"("error in (no error)"=w498, "Parameter"=w496, "Handle in"=w500) -> ("error out"=w497:errorcluster, "Value out"=w495:dbl, "Handle out"=w499:u32)  [unwired: 6 in]
            n354 = local write "Readout Direction"(w495) -> ()
            n355 = call <userlib>:"tm_preparecapture.vi"("error in (no error)"=w497, "Capture mode"=w502, "Handle in"=w499) -> ("error out"=w505:errorcluster, "Buffer Info"=w494:T7, "Handle out"=w508:u32)  [unwired: 5 in, 1 out]
            n356 = call <userlib>:"tm_startcapture_b.vi"("error in (no error)"=w505, "Handle in"=w508) -> ("error out"=w506:errorcluster, "Handle out"=w507:u32)  [unwired: 8 in]
          }
          frame "Disengage Update" {
          }
        }
        n357 = local read "stop"() -> (w121:bool)
        n358 = Compound Arithmetic op=OR(w121, w120) -> (w119:bool)
      }
      n359 = while {
        tunnel: w9 -> [w1039]
        shift-right: [w1035] -> _
        shift-left: _ -> [w1033]
        shift-right: [w1031] -> _
        shift-left: _ -> [w1032]
        shift-right: [w1029] -> _
        shift-left: _ -> [w1025]
        stop <- w1034 stop-if-true
        n360 = Dequeue Element(queue=w1039) -> (element=w1038:T3, timed out?=w1026:bool)  [unwired: 2 in, 2 out]
        n361 = Unbundle By Name(w1038) -> ("State"=w1037:T1, "Stack Number"=w1036:i32, "Image"=w1027:u16[][])
        "State" <- w1037
        n362 = case shown="False" w1026 {
          tunnel: w1027 -> [w1041 w1043]
          tunnel: [w1041 w1042] -> w1028
          tunnel: [w1040 w1043] -> w1029
          tunnel: w1025 -> [w1040 w1042]
          frame False {
          }
          frame True {
          }
        }
        "Image" <- w1028
        n363 = case shown="\"Start Sequence\"" w1037 {
          tunnel: w1036 -> [_ _ _ _ _ _]
          tunnel: [w1046 w1063 _ _ _ _] -> w1035
          tunnel: w1033 -> [_ w1064 w1070 _ _ _]
          tunnel: [FALSE _ _ _ TRUE _] -> w1034
          tunnel: w1028 -> [w1044 w1065 _ _ _ _]
          tunnel: w1032 -> [_ w1062 w1068 w1080 w1105 w1107]
          tunnel: [w1047 w1061 w1069 w1077 w1105 w1107] -> w1031
          tunnel: "Path" -> [w1050 _ _ w1082 _ _]
          frame "Start Sequence" {
            # "Public tiff library"
            # "Get path and open file"
            n364 = Equal?(x=w1050, y=path "") -> (x = y?=w1052:bool)
            n365 = case shown="True" w1052 {
              tunnel: w1050 -> [w1054 _]
              tunnel: [w1054 w1057] -> w1049
              frame False {
              }
              frame True {
                n366 = call "File Dialog"("pattern (all files)"=".tiff", "pattern label"="Tiff Image") -> ("selected path"=w1057:path)  [unwired: 10 in, 3 out]
              }
            }
            n367 = case shown="True" "AutoIncrement" {
              tunnel: w1049 -> [w1058 w1060]
              tunnel: [w1058 w1059] -> w1045
              frame False {
              }
              frame True {
                n368 = call "4Digit File Incrementer.vi"("path"=w1060) -> ("appended path"=w1059:path)  [unwired: 10 in]
              }
            }
            n369 = local write "Path"(w1045) -> ()
            n370 = call-poly "CTIFFNewFileAndStyle.vi"("image"=w1044, "output_file"=w1045) -> ("error"=w1047:errorcluster, "CTIFF"=w1046:i64)  [unwired: 8 in]
          }
          frame "Collecting" {
            # "Add Image to write scan line"
            n371 = call-poly "CTIFFAddNewPage.vi"("error"=w1062, "image"=w1065, "CTIFF"=w1064) -> ("error"=w1061:errorcluster, "CTIFF"=w1063:i64)  [unwired: 7 in]
            n372 = property on="Ram Record" class="Bool (strict)"("DisabledEnum"=T4."Disabled and Grayed Out" ("Disabled"), "BoolText.Text"="Saving" ("Boolean Text.Text")) -> ()  [unwired: 2 in, 2 out]
          }
          frame "End" {
            (unwired) FALSE
            # "Close image file, reset capturing button"
            n373 = call "CTIFFWriteAndClose.vi"("error"=w1068, "CTIFF"=w1070) -> ("error"=w1069:errorcluster)  [unwired: 9 in]
            n374 = property on="Ram Record" class="Bool (strict)"("BoolText.Text"="OK" ("Boolean Text.Text"), "DisabledEnum"=T4."Enabled" ("Disabled")) -> ()  [unwired: 2 in, 2 out]
          }
          frame "Read Disk" {
            w1073 = path "C:/temp.tmp" ("Temp 2")
            # "Can't just send hardisk record in a loop a bunch of times though.\nHave to modify consumer"
            # "This is the easiest option."
            # "Could potentially implments stacks into ram and hardisk record"
            # "For instance the harddisk record may be set to record 5000 images, this could then be used to chunk that into\n50 stacks of 100"
            # "Use stacks one day for rapid imaging , whatevr."
            n375 = call <userlib>:"tm_opendcimgfile.vi"("Path"=w1073) -> ("Total Frames"=w1083:i32, "File Handle"=w1084:u32)  [unwired: 8 in, 1 out]
            n376 = for {
              N: w1083 -> [_]
              tunnel: w1082 -> [w1092]
              shift-right: [w1090] -> w1078
              shift-left: i64 0 ("CTIFF") -> [w1091]
              tunnel: [w1089] -> w1079
              tunnel: w1080 -> [w1088]
              shift-right: [w1094] -> w1074
              shift-left: w1084 -> [w1095]
              i -> [w1085]
              n377 = local write "Stack Frames"(w1085) -> ()
              n378 = Equal To 0?(x=w1085) -> (x = 0?=w1093:bool)
              n379 = call <userlib>:"tm_getdcimgframe.vi"("error in (no error)"=w1088, "Frame Index"=w1085, "File Handle in"=w1095) -> ("error out"=w1087:errorcluster, "Data"=w1086:u16[][], "File Handle out"=w1094:u32)  [unwired: 5 in, 1 out]
              n380 = local write "Image"(w1086) -> ()
              n381 = case shown="True" w1093 {
                tunnel: w1092 -> [_ w1104]
                tunnel: w1086 -> [w1096 w1103]
                tunnel: w1091 -> [w1100 _]
                tunnel: [w1099 w1102] -> w1090
                tunnel: [w1098 w1101] -> w1089
                tunnel: w1087 -> [w1097 _]
                frame False {
                  n382 = call-poly "CTIFFAddNewPage.vi"("error"=w1097, "image"=w1096, "CTIFF"=w1100) -> ("error"=w1098:errorcluster, "CTIFF"=w1099:i64)  [unwired: 7 in]
                }
                frame True {
                  n383 = call-poly "CTIFFNewFileAndStyle.vi"("image"=w1103, "output_file"=w1104) -> ("error"=w1101:errorcluster, "CTIFF"=w1102:i64)  [unwired: 8 in]
                }
              }
            }
            n384 = call "CTIFFWriteAndClose.vi"("error"=w1079, "CTIFF"=w1078) -> ("error"=w1076:errorcluster)  [unwired: 9 in]
            n385 = call <userlib>:"tm_closedcimgfile.vi"("error in (no error)"=w1076, "File Handle"=w1074) -> ("error out"=w1075:errorcluster)  [unwired: 9 in]
            n386 = Delete(path (use dialog)=w1073, error in=w1075) -> (error out=w1077:errorcluster)  [unwired: 3 in, 2 out]
          }
          frame "STOP" {
          }
          frame "Idle" {
          }
        }
      }
      n387 = while {
        tunnel: w10 -> [w91]
        stop <- "stop" stop-if-true
        n388 = event shown="[5] \"Ram Record\": Value Change" {
          selector: _ -> [_ _ _ _ _ _ _ _ _]
          dyn-events: _ -> [_ _ _ _ _ _ _ _ _]
          timeout: _ -> [_ _ _ _ _ _ _ _ _]
          tunnel: w91 -> [_ w93 w95 w96 w98 w101 w106 w112 w115]
          event Timeout {
            n389 = event-data() -> ()  [unwired: 1 in, 3 out]
          }
          event "Camera Readout Mode": Value Change {
            n390 = event-data() -> ()  [unwired: 1 in, 6 out]
            n391 = Enqueue Element(queue=w93, element=CameraControlTypeDef."Readout Mode" ("Enum")) -> ()  [unwired: 2 in, 3 out]
          }
          event "V Width", "V Offset", "H Width", "H Offset": Value Change {
            n392 = event-data() -> ()  [unwired: 1 in, 6 out]
            n393 = Enqueue Element(queue=w95, element=CameraControlTypeDef."ROI" ("Enum")) -> ()  [unwired: 2 in, 3 out]
          }
          event "Readout Direction": Value Change {
            n394 = event-data() -> ()  [unwired: 1 in, 6 out]
            n395 = Enqueue Element(queue=w96, element=CameraControlTypeDef."Readout Direction" ("Enum")) -> ()  [unwired: 2 in, 3 out]
          }
          event "Binning": Value Change {
            n396 = event-data() -> ()  [unwired: 1 in, 6 out]
            n397 = Enqueue Element(queue=w98, element=CameraControlTypeDef."Binning" ("Enum")) -> ()  [unwired: 2 in, 3 out]
          }
          event "Ram Record": Value Change {
            n398 = event-data() -> ("NewVal"=w100:bool)  [unwired: 1 in, 5 out]
            n399 = case shown="True" w100 {
              tunnel: w101 -> [_ w103]
              frame False {
              }
              frame True {
                n400 = Enqueue Element(queue=w103, element=CameraControlTypeDef."Ram Record" ("Enum")) -> ()  [unwired: 2 in, 3 out]
              }
            }
          }
          event "Time Lapse": Value Change {
            n401 = event-data() -> ("NewVal"=w105:bool)  [unwired: 1 in, 5 out]
            n402 = for {
              N: "Stacks" -> [_]
              tunnel: w106 -> [w108]
              tunnel: w105 -> [w107]
              n403 = case shown="True" w107 {
                tunnel: w108 -> [_ w110]
                frame False {
                }
                frame True {
                  n404 = Enqueue Element(queue=w110, element=CameraControlTypeDef."Ram Record" ("Enum")) -> ()  [unwired: 2 in, 3 out]
                }
              }
            }
          }
          event "HardDisk Record": Value Change {
            n405 = event-data() -> ("NewVal"=w111:bool)  [unwired: 1 in, 5 out]
            n406 = case shown="True" w111 {
              tunnel: w112 -> [_ w113]
              frame False {
              }
              frame True {
                n407 = Enqueue Element(queue=w113, element=CameraControlTypeDef."HardDisk Record" ("Enum")) -> ()  [unwired: 2 in, 3 out]
              }
            }
          }
          event "Exposure", "Internal Line Interval", "Trigger Source": Value Change {
            n408 = event-data() -> ()  [unwired: 1 in, 6 out]
            n409 = Enqueue Element(queue=w115, element=CameraControlTypeDef."Update" ("Enum")) -> ()  [unwired: 2 in, 3 out]
          }
        }
      }
      n410 = call <userlib>:"tm_stopcapture.vi"("error in (no error)"=w7, "Handle in"=w8) -> ("error out"=w59:errorcluster, "Handle out"=w60:u32)  [unwired: 8 in]
      n411 = call <userlib>:"tm_unpreparecapture.vi"("error in (no error)"=w59, "Handle in"=w60) -> ("error out"=w58:errorcluster, "Handle out"=w61:u32)  [unwired: 8 in]
      n412 = call <userlib>:"tm_closecamera.vi"("error in (no error)"=w58, "Handle in"=w61) -> ("error out"=w87:errorcluster)  [unwired: 9 in]
      n413 = call <userlib>:"tm_deinitialize.vi"("error in (no error)"=w87) -> ("error out"=w86:errorcluster)  [unwired: 10 in]
    }
  }
  "error out" <- w3
